vi "Motor Controller_Process.vi"(8 "error in":errorcluster, 9 "Process Sync":refnum<notifier>, 10 "TopLevel":refnum<class "TopLevel.lvclass">, 11 "Motor Controller in":refnum<class "Motor Controller.lvclass">) -> (3 "Motor Controller out":refnum<class "Motor Controller.lvclass">)   [LabVIEW 2022 SP3, in "Motor Controller.lvclass"]
uses:
  Motor Controller.lvclass
  TopLevel/TopLevel.lvclass
  Typedefs/Motor Controller Parameter-Set.ctl
  Typedefs/API Event Data.ctl
  Typedefs/API Task State.ctl
  Typedefs/API Command Cluster.ctl
  Typedefs/API Command Enum.ctl
  TopLevel/Typedefs/Motor Controller Config Data.ctl
  Typedefs/Batch Index Speed Data.ctl
  Typedefs/Move Status.ctl
  <vilib>/ethernetip/ethernetip.llb/ethernetip.ctl
  Typedefs/Motor Controller Parameter-Get.ctl
  Typedefs/SetExplicitMessage API Data.ctl
  Typedefs/StageMoves.ctl
  Typedefs/Stage Move Data.ctl
  C:/projects/Digilens_IPLC2/Classes/Motor Controller/EEIP.dll
  EEIP.dll
  <vilib>/ethernetip/ethernetip.lvlib
panel:
  out "error out":errorcluster
  in  "OK":bool
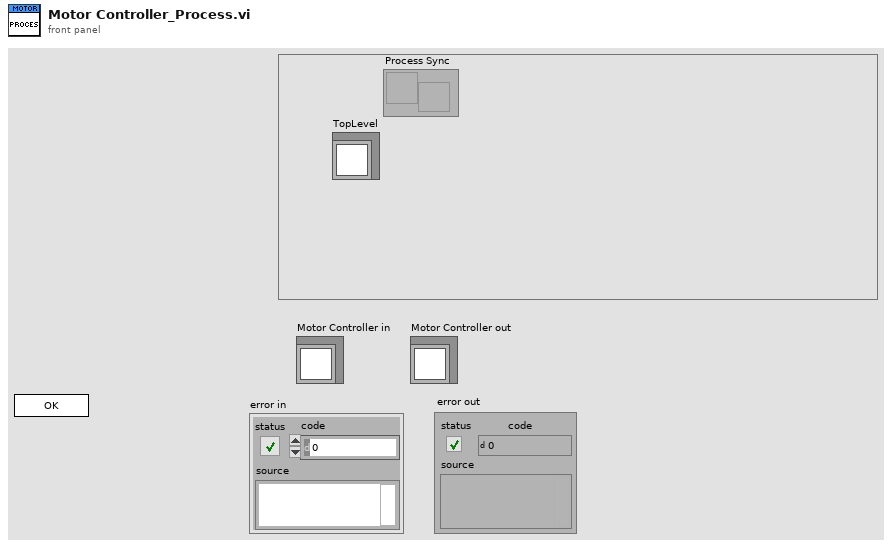
[diagram p1: front panel]
types:
  T1 = typedef "Motor Controller.lvclass/Motor Controller Parameter-Set.ctl" = enum16{"Print Speed", "Jog Speed", "PR Path", "Enable Servo", "Disable Servo", "Move Stage to Under PH1", "Move Stage to Under PH2", "Move Stage to Under PH3", "Move Stage to Under PH4", "Move Stage to Under PH5", "Move Stage to Under PH6", "Home Stage", "Return Stage to 0", "Print Stage", "Write Speed", "Write Index", "Stop Stage"}
  T2 = typedef "Motor Controller.lvclass/API Event Data.ctl" = cluster{"Task":cluster{"Time Stamp":timestamp, "Timeout (ms)":u32, "Task State":T3, "Task Error":errorcluster, "Task ID":string}, "Command":variant, "Return Value":variant}
  T3 = typedef "Motor Controller.lvclass/API Task State.ctl" = enum16{"Completed", "Errored", "Pending"}
  T4 = typedef "Motor Controller.lvclass/API Command Cluster.ctl" = cluster{"Command":T5, "Arguments":string, "Data":variant}
  T5 = typedef "Motor Controller.lvclass/API Command Enum.ctl" = enum16{"GetExplicitMessage", "SetExplicitMessage", "Execute Stage Move Recipe", "Read Stage Move Recipe", "Abort"}
  T6 = enum32{"invalid app kind", "Development System", "Run Time System", "Student Edition", "Embedded LabVIEW", "Evaluation", "Custom"}
  T7 = enum32{"Invalid", "Standard", "Closed", "Hidden", "Minimized", "Maximized"}
  T8 = typedef "Motor Controller.lvclass/Motor Controller Parameter-Get.ctl" = enum16{"Print Speed", "Jog Speed", "PR Path", "Servo Enabled?", "AlarmCodes"}
  T9 = typedef "Motor Controller.lvclass/SetExplicitMessage API Data.ctl" = cluster{"Motor Controller Parameter":T1, "value":i32}
  T10 = typedef "Motor Controller.lvclass/Stage Move Data.ctl" = cluster{"Current Step":string, "Move Data":T11[]}
  T11 = typedef "Motor Controller.lvclass/Batch Index Speed Data.ctl" = cluster{"Batch & Cycle":string, "Move":cluster{"Index_mm":i32, "Speed_mm_s":i32}, "Status":T12}
  T12 = typedef "Motor Controller.lvclass/Move Status.ctl" = enum16{"Pending", "In Progress", "Completed"}
  T13 = cluster{"Time Stamp":timestamp, "Timeout (ms)":u32, "Task State":T3, "Task Error":errorcluster, "Task ID":string}
  T14 = typedef "Motor Controller.lvclass/Motor Controller Config Data.ctl" = cluster{"Motor IP Addresss":string, "Current Position":i32, "Pulse_Per_mm":i32, "PrePrint":dbl[], "Load Position_mm":i32, "Laminate Position_mm":i32}
  T15 = typedef "TopLevel.lvclass/Digilens Config Cluster.ctl" = cluster{"Motion Controller":T14, "IO Config":T16, "PrinterConfiguration":T19, "DAQ Settings":T20}
  T16 = typedef "IO.lvclass/IO Config Data.ctl" = cluster{"DAQDevices":T17[], "DI Channels":T18[], "DO Channels":T18[], "Material Names":string[], "AI Channels":T18[], "AO Channels":T18[]}
  T17 = typedef "IO.lvclass/DCON_DeviceConfig--Cluster.ctl" = cluster{"COM":string, "DeviceName":string, "BaudRate":u32, "Number of Channels":i32, "DeviceAddress":i32, "Enable":bool}
  T18 = typedef "IO.lvclass/Channel Data.ctl" = cluster{"Channel Name":string, "Device Name":string, "Channel No":string}
  T19 = typedef "GIS Printer.lvclass/PrinterConfiguration--Cluster.ctl" = cluster{"IPAddress":string, "Move Stage on RTP Command?":bool, "Stage Move Position":string, "PH1-Prime Path":path, "PH2-Prime Path":path, "PH3-Prime Path":path, "PH4-Prime Path":path, "PH5-Prime Path":path, "PH6-Prime Path":path, "PrintScriptsFolder":path, "PurgeScriptsFolder":path, "StageScriptsFolder":path, "PH1-HeatOn Path":path, "PH2-HeatOn Path":path, "PH3-HeatOn Path":path, "PH4-HeatOn Path":path, "PH5-HeatOn Path":path, "PH6-HeatOn Path":path, "PH1-HeatOff Path":path, "PH2-HeatOff Path":path, "PH3-HeatOff Path":path, "PH4-HeatOff Path":path, "PH5-HeatOff Path":path, "PH6-HeatOff Path":path}
  T20 = typedef "DAQ.lvclass/TD DAQ Settings--cluster.ctl" = cluster{"Simulate DAQ":bool, "DI Settings":T21[], "AI Settings":T22[], "Relay IONames":string[], "AO IONames":string[], "AO NChan SingleTask":bool}
  T21 = typedef "DAQ.lvclass/TD DI Instrument Settings--cluster.ctl" = cluster{"Disable":bool, "DI TaskName":string, "DI RefreshIntv":i32}
  T22 = typedef "DAQ.lvclass/TD AI Instrument Settings--cluster.ctl" = cluster{"Disable":bool, "AI TaskName":string, "AI InstSettings":T23, "SimAI Ranges":T24}
  T23 = typedef "DAQ.lvclass/TD AI InstSettings--cluster.ctl" = cluster{"DaqRate":dbl, "NumSamples":i32}
  T24 = typedef "DAQ.lvclass/TD SimAI Ranges--cluster.ctl" = cluster{"lo":dbl, "hi":dbl}
  T25 = typedef "ethernetip.lvlib/ethernetip.ctl" = refnum<k21>
  T26 = cluster{"Core":cluster{"Current VI Reference":refnum<vi>, "Close Panel on Exit?":bool}, "Motor Controller out":refnum<class "Motor Controller.lvclass">, "Tasks":T2[], "TO":i32, "API Executed Event":refnum<user-event>, "API Return Event":refnum<user-event>, "Current Task":T4, "Task Start ms":u32, ".NET Refnum":refnum<k24>, "Current Task. Return Value":variant, "Motion Controller Config Data":T14, "Methods:Accessors:Digilens Config":T15, "Stage Moves":T11[], "Move Index":i32, "Session out":T25, "Process Sync":refnum<notifier>}
  T27 = cluster{"Current VI Reference":refnum<vi>, "Close Panel on Exit?":bool}
  T28 = typedef "Motor Controller.lvclass/UserEvents.ctl" = cluster{"API Incoming Event":refnum<user-event>, "API Executed Event":refnum<user-event>, "API Return Event":refnum<user-event>, "Status Changed Event":refnum<user-event>, "StopEvent":refnum<user-event>}
  T29 = typedef "TopLevel.lvclass/UserEvents.ctl" = cluster{"API Incoming Event":refnum<user-event>, "API Executed Event":refnum<user-event>, "API Return Event":refnum<user-event>, "Exit Event":refnum<user-event>, "StatusChanged":refnum<user-event>, "DLP GUI Config Changed":refnum<user-event>, "AppEvent":refnum<user-event>, "Login Event":refnum<user-event>, "HeadPrimeStatusEvent":refnum<user-event>}
  T30 = typedef "Motor Controller.lvclass/StageMoves.ctl" = cluster{"Batch_Move":cluster{"Cycles":u32, "Move":cluster{"Index_mm":i32, "Speed_mm_s":i32}[]}[]}
  T31 = cluster{"Cycles":u32, "Move":cluster{"Index_mm":i32, "Speed_mm_s":i32}[]}[]
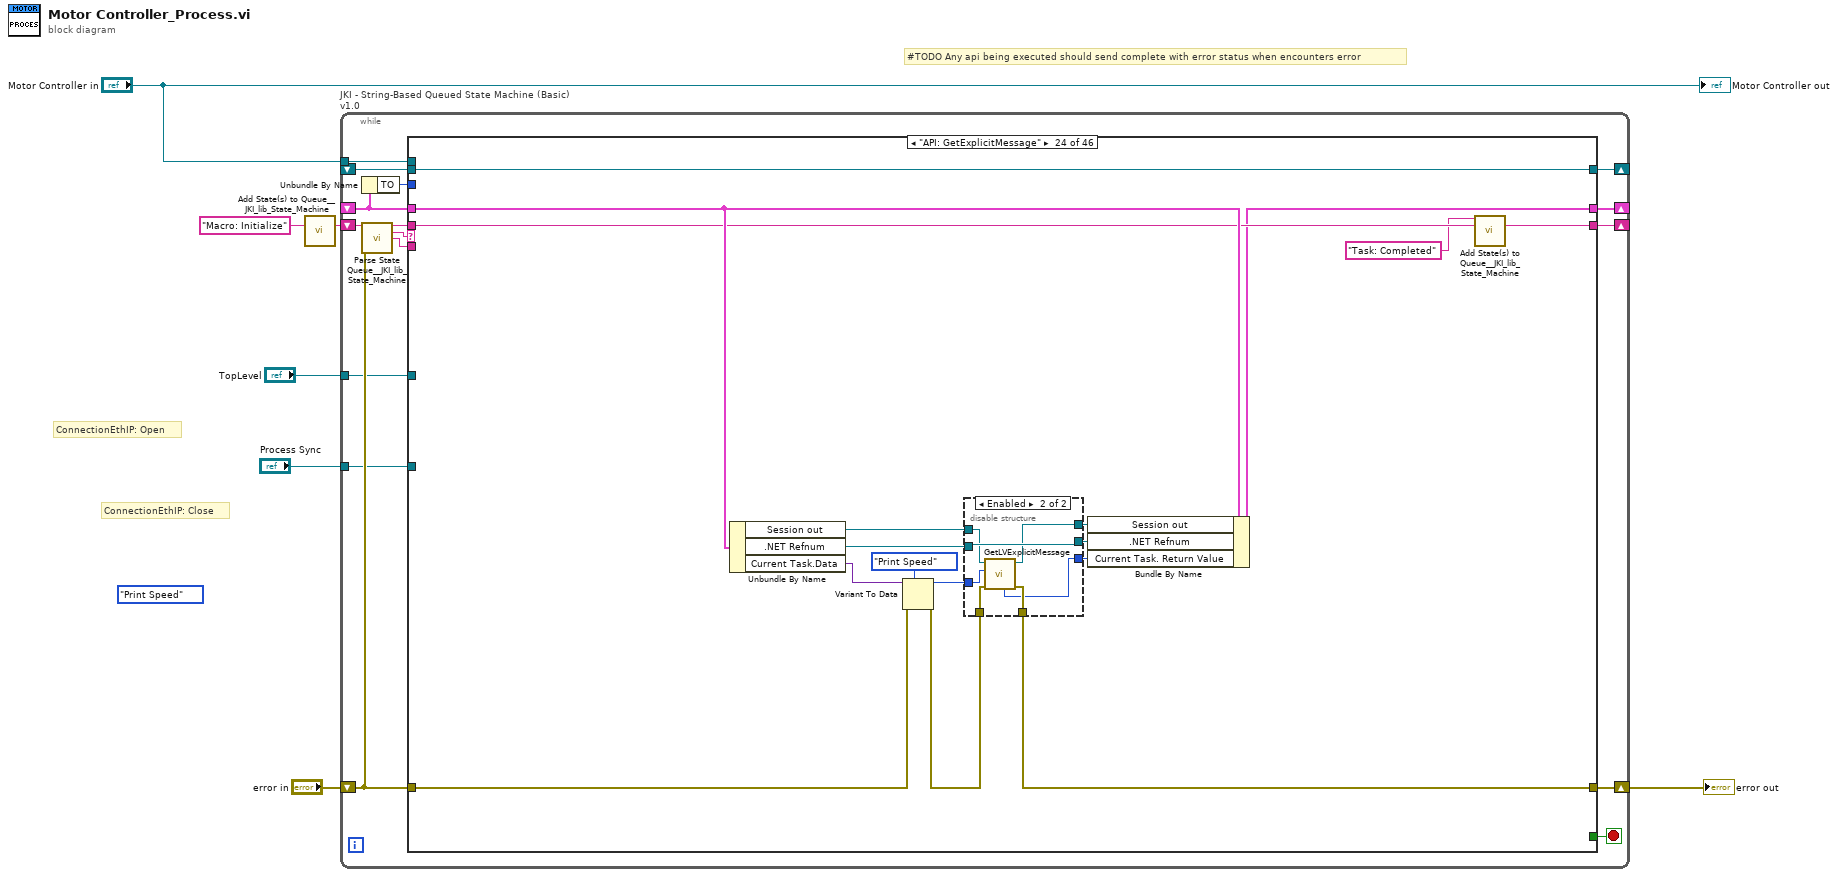
[diagram p0: block diagram]
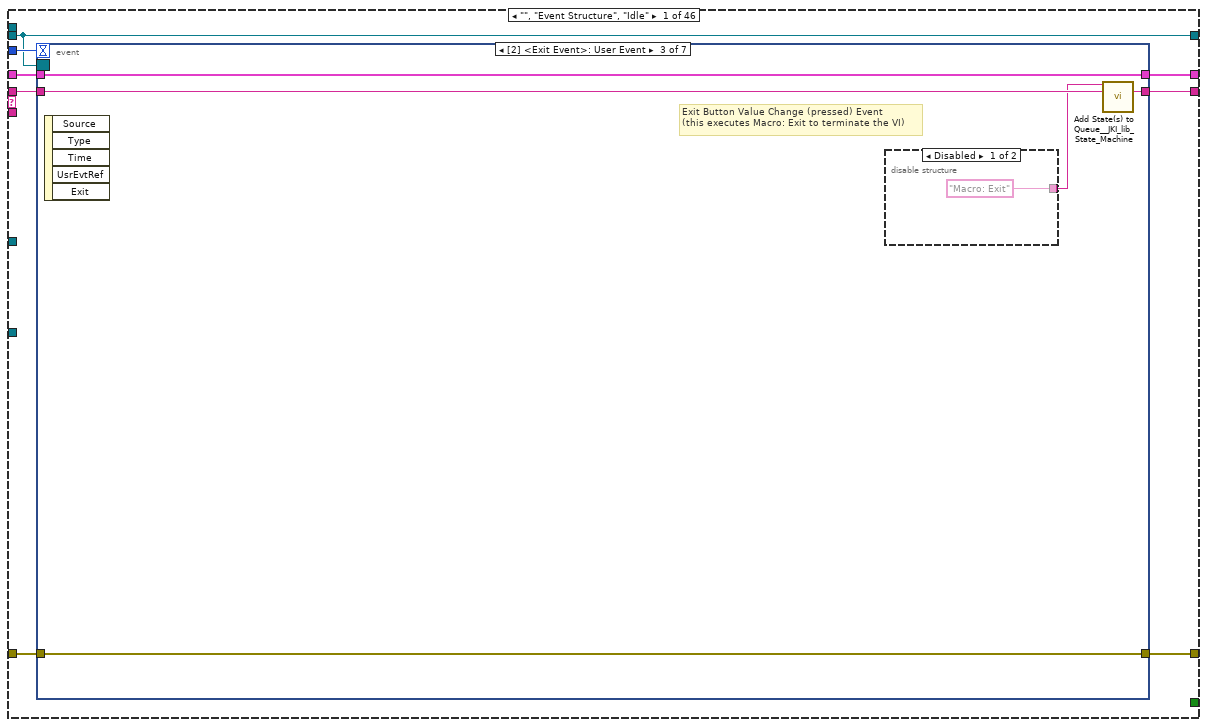
[diagram p2: hidden frame]
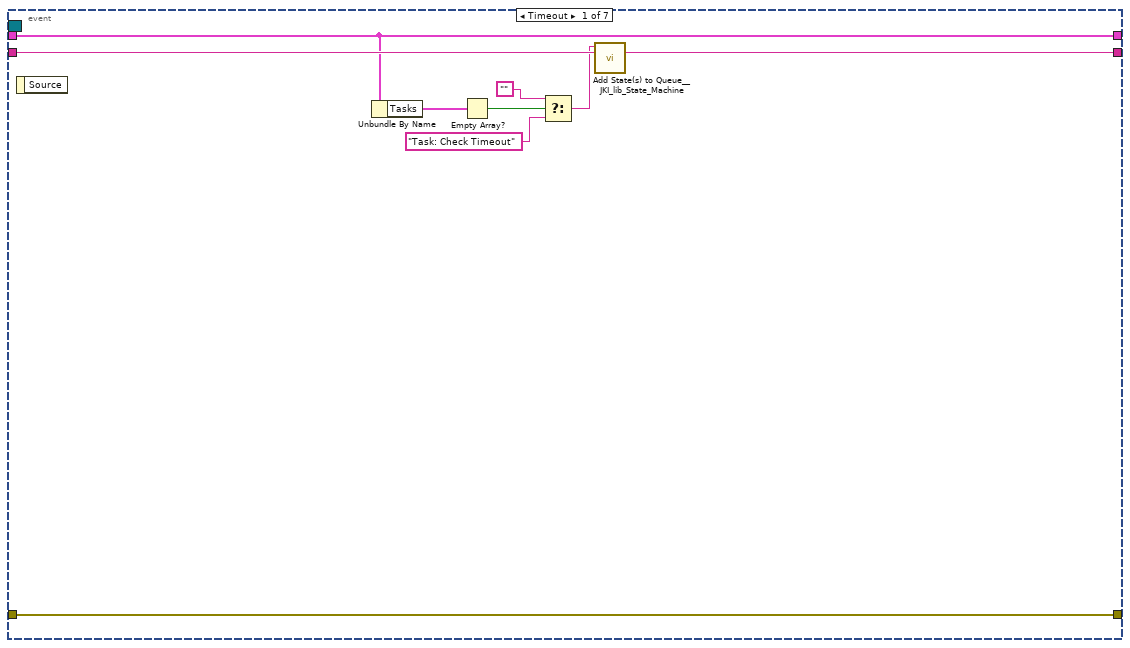
[diagram p3: hidden frame]
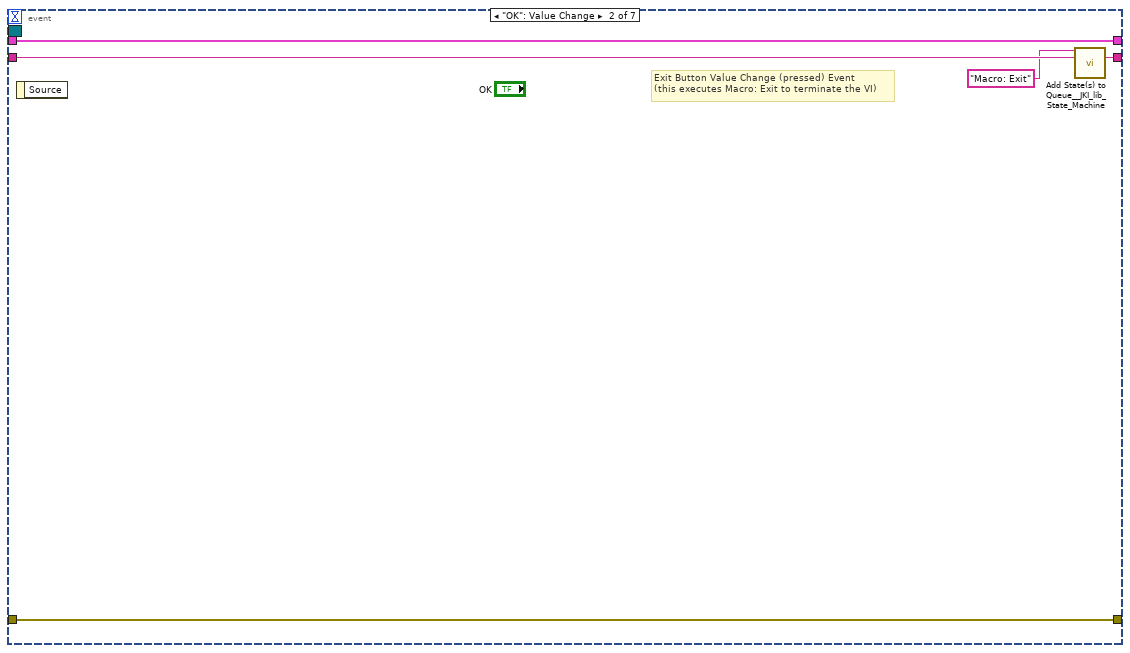
[diagram p4: hidden frame]
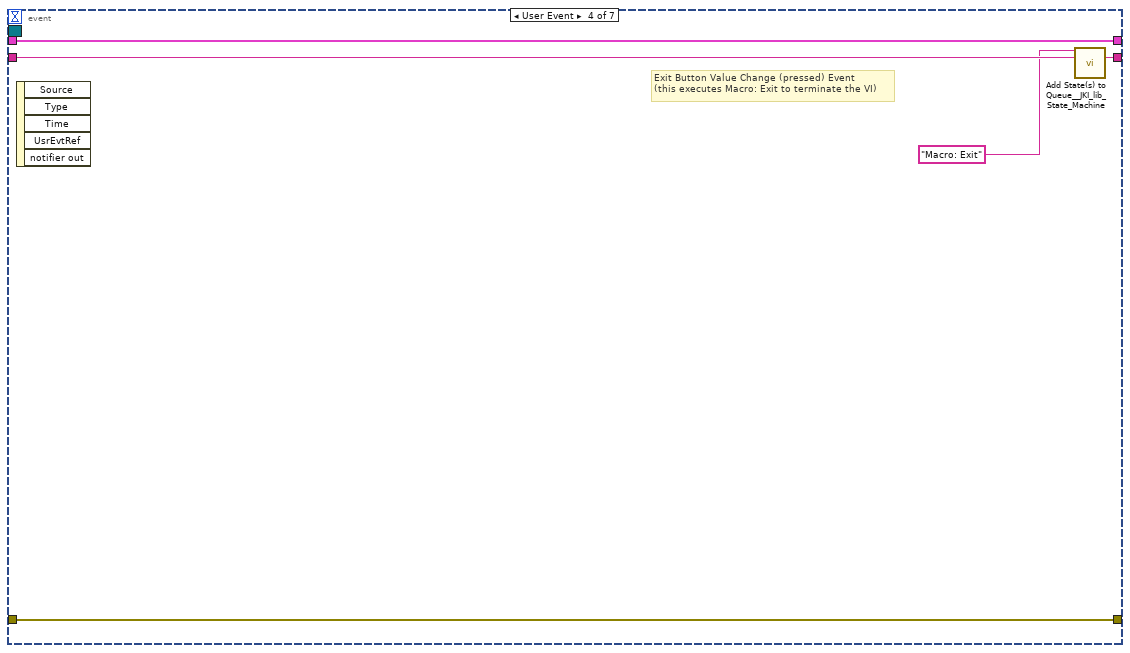
[diagram p6: hidden frame]
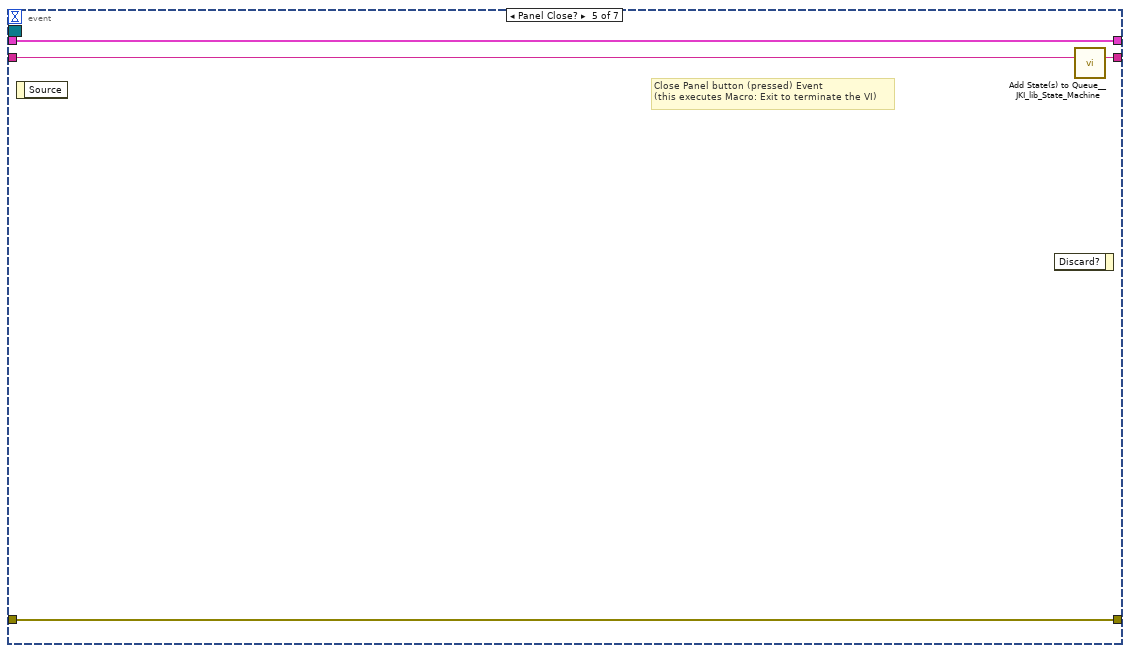
[diagram p7: hidden frame]
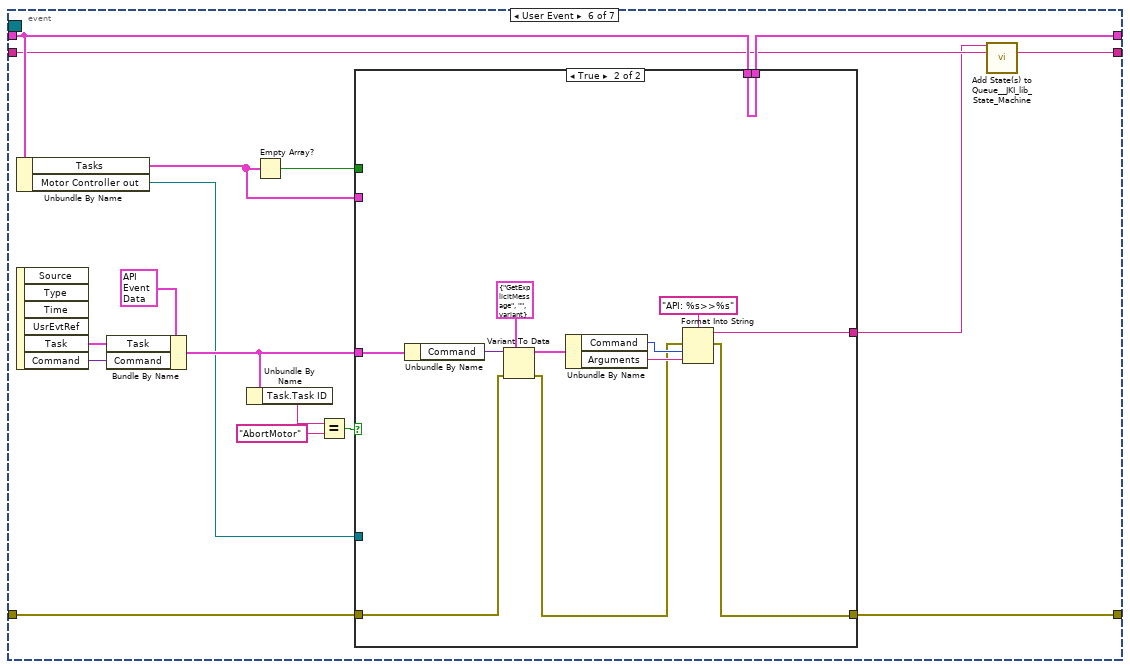
[diagram p8: hidden frame]
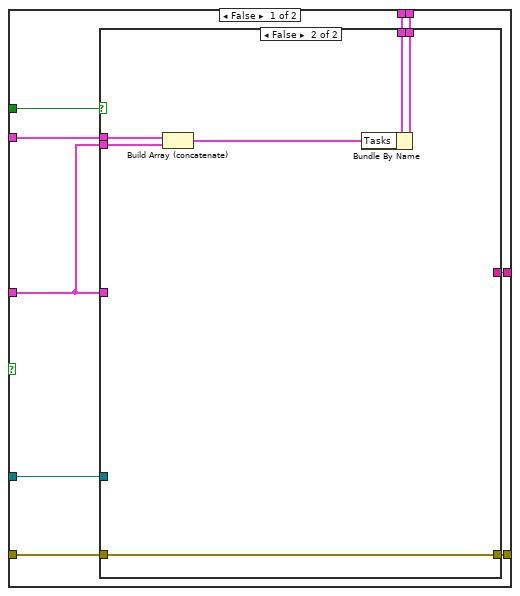
[diagram p9: hidden frame]
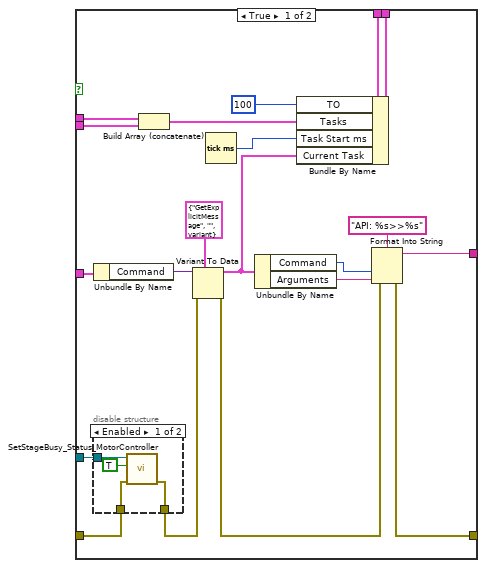
[diagram p10: hidden frame]
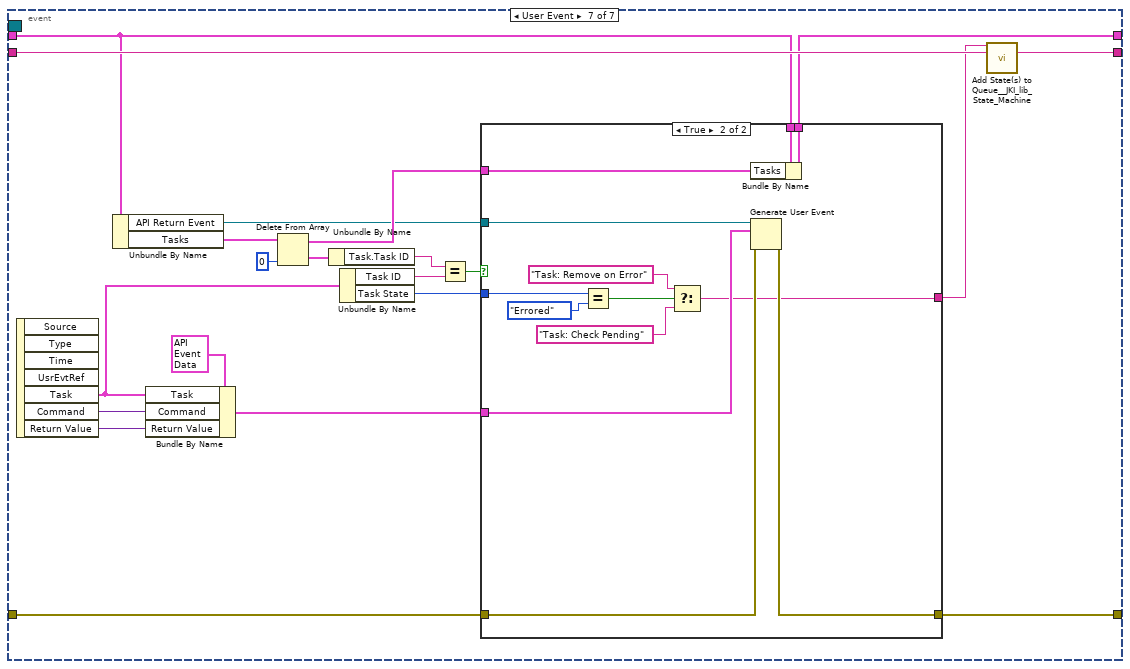
[diagram p12: hidden frame]
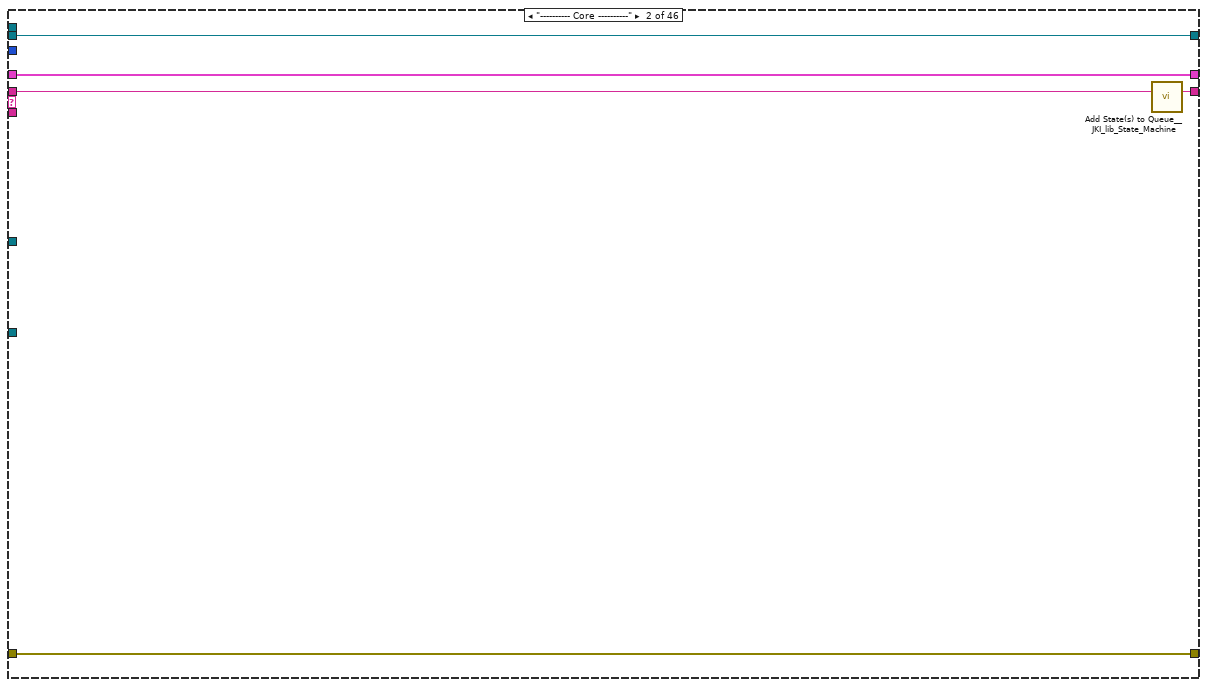
[diagram p14: hidden frame]
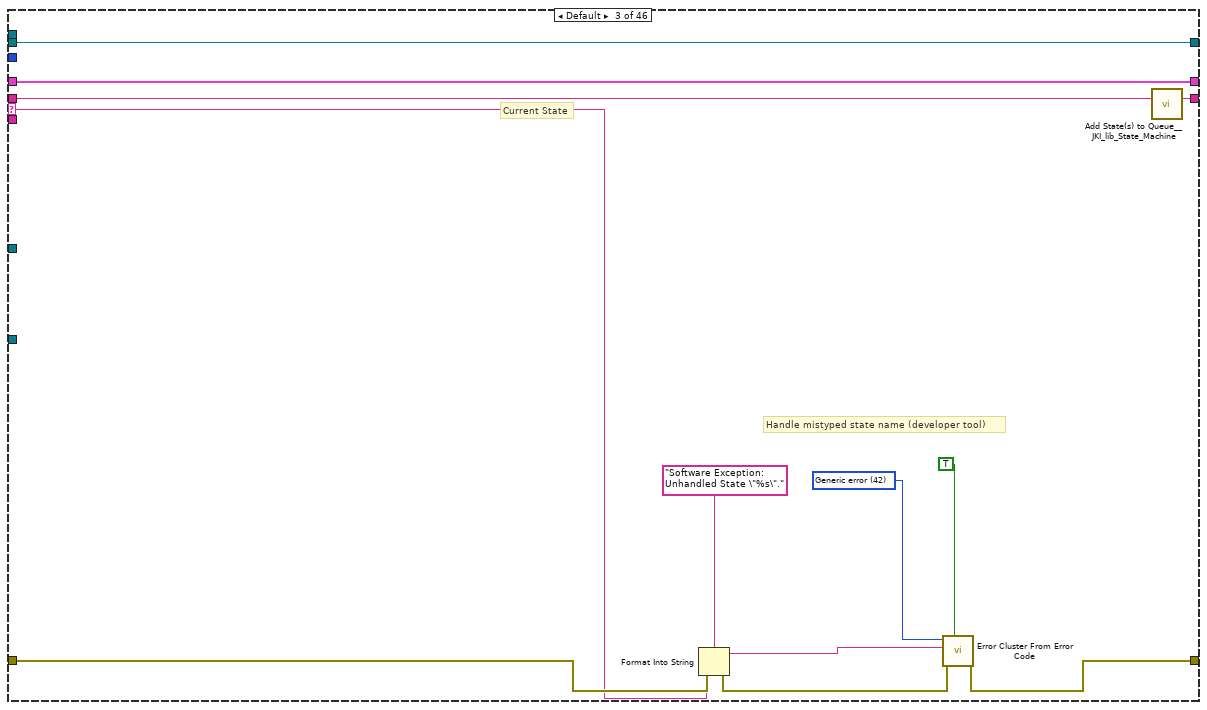
[diagram p15: hidden frame]
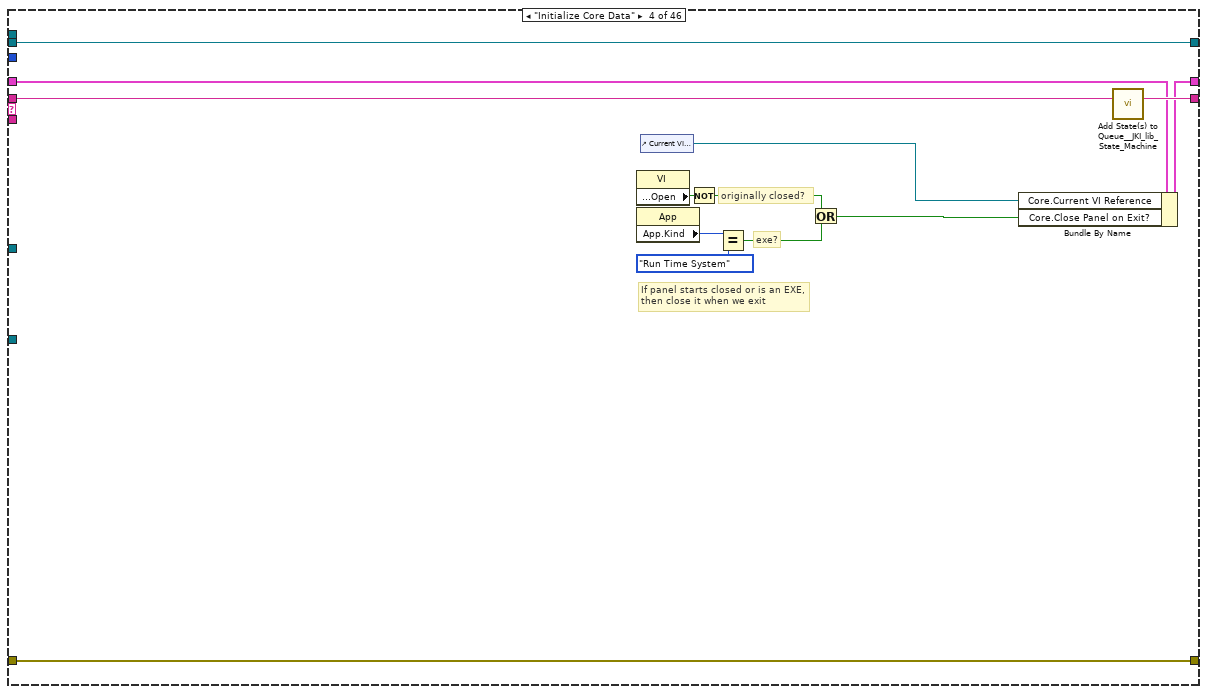
[diagram p16: hidden frame]
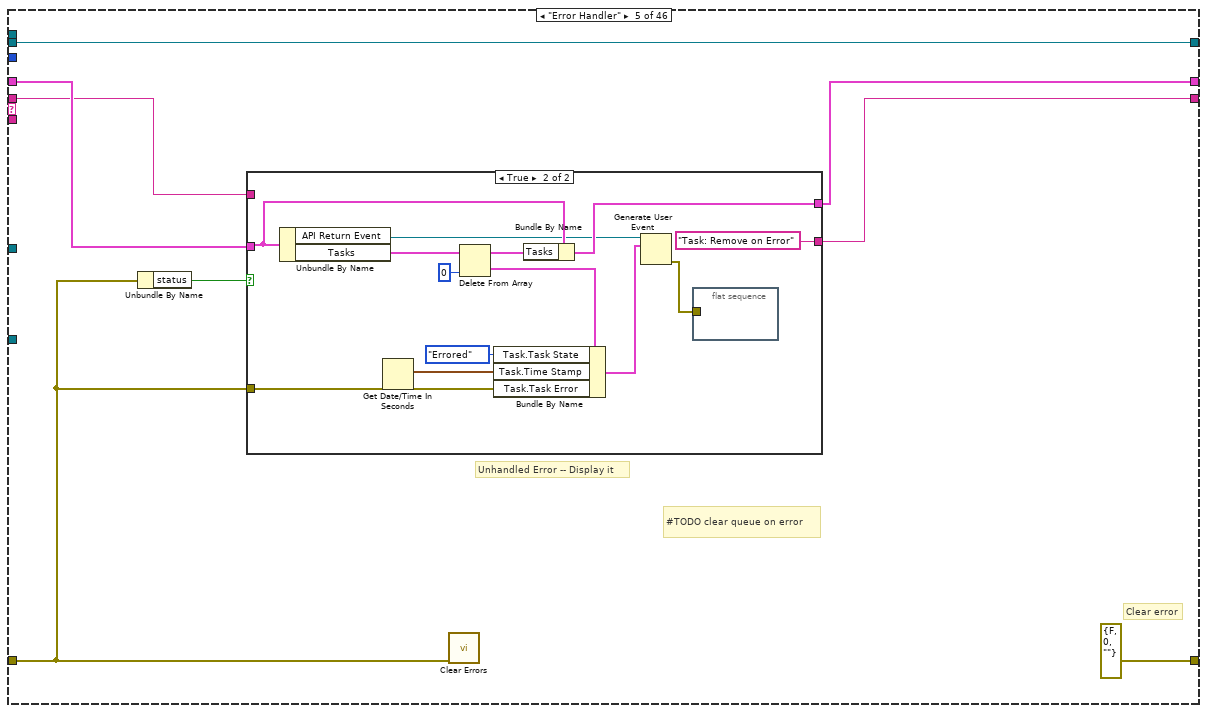
[diagram p17: hidden frame]
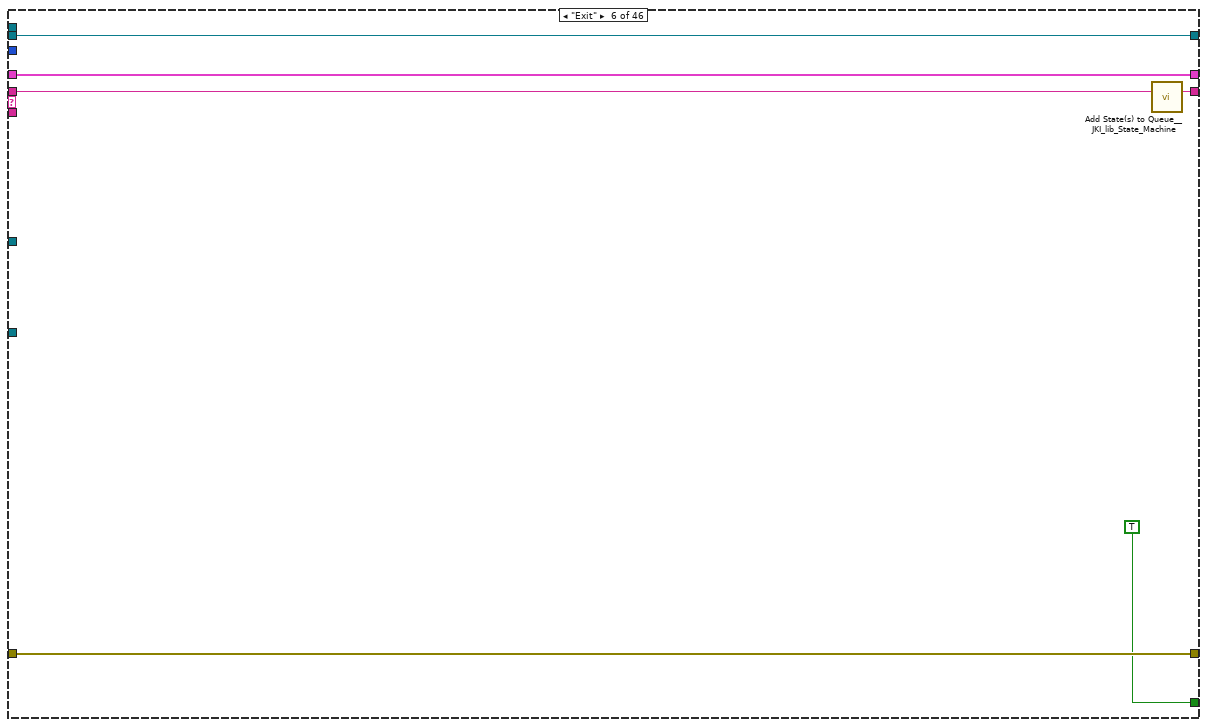
[diagram p19: hidden frame]
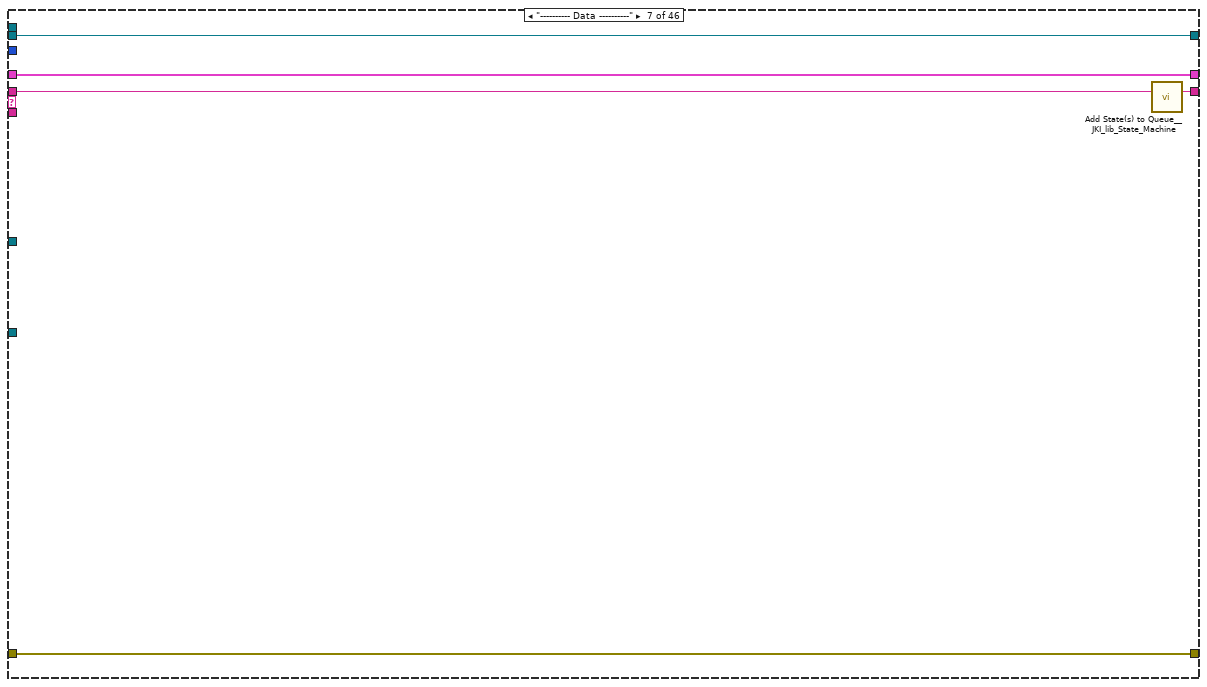
[diagram p20: hidden frame]
diagram:
  (unwired) Motor_Controller_Parameter-Set."Print Speed" ("Motor Controller Parameter")
  # "ConnectionEthIP: Close"
  # "ConnectionEthIP: Open"
  # "#TODO Any api being executed should send complete with error status when encounters error"
  n1 = call <vilib>:"Add State(s) to Queue__JKI_lib_State_Machine.vi"("State(s) in (\"\")"="Macro: Initialize") -> ("States Out"=w7:string)  [unwired: 14 in]
  n2 = while "JKI - String-Based Queued State Machine (Basic) v1.0" {
    shift-right: [w16] -> _
    shift-left: _ -> [w10]
    shift-right: [w19] -> w3
    shift-left: "error in" -> [w15]
    shift-right: [w18] -> _
    shift-left: w7 -> [w20]
    tunnel: "Motor Controller in" -> [w14]
    shift-right: [w13] -> _
    shift-left: _ -> [w12]
    tunnel: "TopLevel" -> [w9]
    tunnel: "Process Sync" -> [w8]
    stop <- w17 stop-if-true
    n3 = Unbundle By Name(w10) -> ("TO"=w11:i32)
    n4 = call <vilib>:"Parse State Queue__JKI_lib_State_Machine.vi"("State Queue"=w20, "Error In (no error)"=w15) -> ("Remaining States"=w22:string, "Current State"=w23:string, "Arguments"=w21:string)  [unwired: 11 in]
    n5 = case shown="\"API: GetExplicitMessage\"" w23 {
      selector: w23 -> [_ _ w172 _ _ _ _ _ _ _ _ _ _ _ _ _ _ _ _ _ _ _ _ _ _ _ _ _ _ _ _ _ _ _ _ _ _ _ _ _ _ _ _ _ _ _]
      tunnel: w22 -> [w31 w170 w176 w195 w196 w224 w229 w237 w263 w272 w277 w283 w290 w302 w329 _ w345 w347 w355 w371 w377 w379 _ w398 w435 w475 w500 w512 w520 w531 w551 w580 w624 w641 w650 w656 w664 w671 w674 w686 w700 w703 w773 w859 w866 w895]
      tunnel: w21 -> [_ _ _ _ _ _ _ _ _ _ _ _ w285 w296 _ _ _ _ _ _ _ _ _ _ _ _ _ _ _ _ _ _ _ _ _ _ _ _ _ _ _ w721 _ _ _ _]
      tunnel: w10 -> [w29 w167 w174 w186 w198 w222 w226 w234 _ w268 w274 w281 w288 w298 w326 w331 w342 w350 w353 w368 w375 w380 w383 w407 w441 w479 w505 w517 w521 w529 w549 w577 w621 w640 w643 w653 w663 w667 w673 w684 w699 w709 w771 w857 w878 w897]
      tunnel: [w28 w168 w178 w192 errorcluster {"status"=FALSE, "code"=0, "source"=""} ("error out") w221 w227 w231 w244 w269 w275 w278 w286 w299 w327 w334 w343 w351 w354 w366 w373 w378 w387 w405 w426 w469 w496 w508 w519 w525 w546 w585 w615 w642 w646 w652 w660 w668 w675 w682 w701 w711 w749 w849 w875 w904] -> w19
      tunnel: w15 -> [w27 w168 w177 w192 w200 w221 w227 w230 w257 w264 w275 w279 w287 w300 w327 w334 w343 w351 w354 w361 w374 w378 w388 w400 w437 w477 w503 w515 w519 w524 w545 w584 w620 w642 w645 w651 w665 w669 w675 w681 w701 w719 w755 w850 w874 w904]
      tunnel: [w30 w169 w175 w194 w197 w223 w228 w236 w263 w271 w276 w282 w289 w301 w328 w333 w344 w348 w355 w370 w376 w379 "Task: Remove on Error" ("State(s) at Back (\"\")") w399 w436 w476 w501 w513 w520 w531 w551 w581 w625 w641 w650 w656 w664 w671 w674 w686 w700 w704 w773 w859 w867 w896] -> w18
      tunnel: [_ _ _ _ _ TRUE _ _ _ _ _ _ _ _ _ _ _ _ _ _ _ _ _ _ _ _ _ _ _ _ _ _ _ _ _ _ _ _ _ _ _ _ _ _ _ _] -> w17
      tunnel: [w26 w167 w174 w193 w199 w222 w226 w234 w262 w268 w274 w281 w288 w298 w326 w331 w342 w350 w353 w358 w375 w380 w384 w396 w434 w474 w505 w517 w521 w529 w549 w578 w619 w640 w644 w653 w658 w667 w673 w677 w699 w710 w758 w852 w878 w898] -> w16
      tunnel: w11 -> [w25 _ _ _ _ _ _ _ _ _ _ _ _ _ _ _ _ _ _ _ _ _ _ _ _ _ _ _ _ _ _ _ _ _ _ _ _ _ _ _ _ _ _ _ _ _]
      tunnel: w14 -> [_ _ _ _ _ _ _ _ w239 _ _ _ _ _ _ _ _ _ _ _ _ _ _ _ _ _ _ _ _ _ _ _ _ _ _ _ _ _ _ _ _ _ _ _ _ _]
      tunnel: [w24 w166 w171 w183 w202 w219 w225 w235 w260 w267 w273 w280 w284 w295 w325 w330 w335 w349 w352 w369 w372 w381 w391 w408 w442 w480 w506 w518 w522 w530 w550 w588 w626 w639 w649 w655 w662 w670 w672 w685 w698 w722 w772 w858 w879 w903] -> w13
      tunnel: w12 -> [w24 w166 w171 w183 w202 w219 w225 w235 w260 w267 w273 w280 w284 w295 w325 w330 w335 w349 w352 _ w372 w381 w391 w408 w442 w480 w506 w518 w522 w530 w550 w588 w626 w639 w649 w655 w662 w670 w672 w685 w698 w722 w772 w858 w879 w903]
      tunnel: w9 -> [_ _ _ _ _ _ _ _ w242 _ _ _ _ _ _ _ _ _ _ w363 _ _ _ _ _ _ _ _ _ _ _ _ _ _ _ _ _ _ _ _ _ _ _ _ _ _]
      tunnel: w8 -> [_ _ _ _ _ _ _ _ w238 _ _ _ _ _ _ _ _ _ _ _ _ _ _ _ _ _ _ _ _ _ _ _ _ _ _ _ _ _ _ _ _ _ _ _ _ _]
      frame "", "Event Structure", "Idle" {
        n6 = event shown="[2] <Exit Event>: User Event" {
          selector: w24 -> [_ _ _ _ _ _ _]
          dyn-events: _ -> [_ _ _ _ _ _ _]
          timeout: w25 -> [_ _ _ _ _ _ _]
          tunnel: w31 -> [w40 w45 w50 w56 w60 w67 w149]
          tunnel: [w39 w44 w49 w55 w59 w68 w150] -> w30
          tunnel: w29 -> [w37 w42 w47 w53 w57 w71 w148]
          tunnel: [w38 w43 w48 w54 w58 w70 w142] -> w28
          tunnel: w27 -> [w38 w43 w48 w54 w58 w69 w143]
          tunnel: [w37 w42 w47 w53 w57 w72 w145] -> w26
          event Timeout {
            n7 = event-data() -> ()  [unwired: 1 in, 1 out]
            n8 = Unbundle By Name(w37) -> ("Tasks"=w36:T2[])
            n9 = Empty Array?(array=w36) -> (empty?=w35:bool)
            n10 = Select(t="", s=w35, f="Task: Check Timeout") -> (s? t:f=w32:string)
            n11 = call <vilib>:"Add State(s) to Queue__JKI_lib_State_Machine.vi"("State(s) in Front (\"\")"=w32, "State(s) in (\"\")"=w40) -> ("States Out"=w39:string)  [unwired: 13 in]
          }
          event "OK": Value Change {
            # "Exit Button Value Change (pressed) Event\n(this executes Macro: Exit to terminate the VI)"
            n12 = event-data() -> ()  [unwired: 1 in, 1 out]
            n13 = call <vilib>:"Add State(s) to Queue__JKI_lib_State_Machine.vi"("State(s) in Front (\"\")"="Macro: Exit", "State(s) in (\"\")"=w45) -> ("States Out"=w44:string)  [unwired: 13 in]
          }
          event User Event {
            # "Exit Button Value Change (pressed) Event\n(this executes Macro: Exit to terminate the VI)"
            n14 = event-data() -> ()  [unwired: 1 in, 5 out]
            n15 = disable-structure shown="Disabled" {
              disable-tunnel: ["Macro: Exit" _] -> w46
              frame Disabled {
              }
              frame Enabled {
              }
            }
            n16 = call <vilib>:"Add State(s) to Queue__JKI_lib_State_Machine.vi"("State(s) in Front (\"\")"=w46, "State(s) in (\"\")"=w50) -> ("States Out"=w49:string)  [unwired: 13 in]
          }
          event User Event {
            # "Exit Button Value Change (pressed) Event\n(this executes Macro: Exit to terminate the VI)"
            n17 = event-data() -> ()  [unwired: 1 in, 5 out]
            n18 = call <vilib>:"Add State(s) to Queue__JKI_lib_State_Machine.vi"("State(s) in Front (\"\")"="Macro: Exit", "State(s) in (\"\")"=w56) -> ("States Out"=w55:string)  [unwired: 13 in]
          }
          event Panel Close? {
            # "Close Panel button (pressed) Event\n(this executes Macro: Exit to terminate the VI)"
            n19 = event-data() -> ()  [unwired: 1 in, 1 out]
            n20 = event-data() -> ()  [unwired: 2 in, 1 out]
            n21 = call <vilib>:"Add State(s) to Queue__JKI_lib_State_Machine.vi"("State(s) in (\"\")"=w60) -> ("States Out"=w59:string)  [unwired: 14 in]
          }
          event User Event {
            n22 = Unbundle By Name(w71) -> ("Tasks"=w73:T2[], "Motor Controller out"=w61:refnum<class "Motor Controller.lvclass">)
            n23 = event-data() -> ("Task"=w76:T13, "Command"=w75:variant)  [unwired: 1 in, 4 out]
            n24 = Bundle By Name(cluster=T2 {"Task"={"Time Stamp"=timestamp(0 s since 1904-01-01), "Timeout (ms)"=0, "Task State"=enum."Completed", "Task Error"={"status"=FALSE, "code"=0, "source"=""}, "Task ID"=""}, "Command"=variant, "Return Value"=variant} ("API Event Data"), "Task"=w76, "Command"=w75) -> (w65:T2)
            n25 = Unbundle By Name(w65) -> ("Task.Task ID"=w64:string)
            n26 = Empty Array?(array=w73) -> (empty?=w74:bool)
            n27 = Equal?(x=w64, y="AbortMotor") -> (x = y?=w62:bool)
            n28 = case shown="True" w62 {
              tunnel: w74 -> [w86 _]
              tunnel: w73 -> [w85 _]
              tunnel: [w84 w129] -> w72
              tunnel: w71 -> [w83 w129]
              tunnel: [w82 w118] -> w70
              tunnel: w69 -> [w81 w120]
              tunnel: [w80 w121] -> w66
              tunnel: w65 -> [w79 w122]
              tunnel: w61 -> [w78 _]
              frame False {
                n29 = case shown="False" w86 {
                  tunnel: w85 -> [w106 w117]
                  tunnel: w79 -> [w105 w116]
                  tunnel: w83 -> [w104 w115]
                  tunnel: [w102 w113] -> w84
                  tunnel: w79 -> [w101 _]
                  tunnel: w81 -> [w87 w112]
                  tunnel: [w97 w112] -> w82
                  tunnel: [w94 _] -> w80
                  tunnel: w78 -> [w89 _]
                  frame True {
                    n30 = Unbundle By Name(w101) -> ("Command"=w100:variant)
                    n31 = disable-structure shown="Enabled" {
                      disable-tunnel: w89 -> [w110 _]
                      disable-tunnel: [w108 w111] -> w88
                      disable-tunnel: w87 -> [w107 w111]
                      frame Enabled {
                        n32 = call "SetStageBusy_Status_MotorController.vi"("error in (no error)"=w107, "Stage Busy?"=TRUE, "Motor Controller in"=w110) -> ("error out"=w108:errorcluster)  [unwired: 7 in, 1 out]
                      }
                      frame Disabled {
                      }
                    }
                    n33 = Build Array (concatenate)(w106, w105) -> (w103:T2[])
                    n34 = Variant To Data(error in=w88, type=T4 {"Command"=enum."GetExplicitMessage", "Arguments"="", "Data"=variant} ("API Command Cluster"), Variant=w100) -> (data=w90:T4, error out=w98:errorcluster)
                    n35 = Tick Count (ms)() -> (millisecond timer value=w92:u32)
                    n36 = Unbundle By Name(w90) -> ("Command"=w95:T5, "Arguments"=w93:string)
                    n37 = Bundle By Name(cluster=w104, "TO"=100, "Tasks"=w103, "Task Start ms"=w92, "Current Task"=w90) -> (w102:T26)
                    n38 = Format Into String(format string="API: %s>>%s", error in=w98, w95, w93) -> (resulting string=w94:string, error out=w97:errorcluster)  [unwired: 1 in]
                  }
                  frame False {
                    n39 = Build Array (concatenate)(w117, w116) -> (w114:T2[])
                    n40 = Bundle By Name(cluster=w115, "Tasks"=w114) -> (w113:T26)
                  }
                }
              }
              frame True {
                n41 = Unbundle By Name(w122) -> ("Command"=w128:variant)
                n42 = Variant To Data(error in=w120, type=T4 {"Command"=enum."GetExplicitMessage", "Arguments"="", "Data"=variant} ("API Command Cluster"), Variant=w128) -> (data=w123:T4, error out=w119:errorcluster)
                n43 = Unbundle By Name(w123) -> ("Command"=w125:T5, "Arguments"=w124:string)
                n44 = Format Into String(format string="API: %s>>%s", error in=w119, w125, w124) -> (resulting string=w121:string, error out=w118:errorcluster)  [unwired: 1 in]
              }
            }
            n45 = call <vilib>:"Add State(s) to Queue__JKI_lib_State_Machine.vi"("State(s) in Front (\"\")"=w66, "State(s) in (\"\")"=w67) -> ("States Out"=w68:string)  [unwired: 13 in]
          }
          event User Event {
            n46 = event-data() -> ("Task"=w136:T13, "Command"=w140:variant, "Return Value"=w139:variant)  [unwired: 1 in, 4 out]
            n47 = Unbundle By Name(w148) -> ("API Return Event"=w133:refnum<user-event>, "Tasks"=w147:T2[])
            n48 = Bundle By Name(cluster=T2 {"Task"={"Time Stamp"=timestamp(0 s since 1904-01-01), "Timeout (ms)"=0, "Task State"=enum."Completed", "Task Error"={"status"=FALSE, "code"=0, "source"=""}, "Task ID"=""}, "Command"=variant, "Return Value"=variant} ("API Event Data"), "Task"=w136, "Command"=w140, "Return Value"=w139) -> (w138:T2)
            n49 = Delete From Array(array=w147, index=0) -> (deleted portion=w137:T2, array with subset deleted=w144:T2[])  [unwired: 1 in]
            n50 = Unbundle By Name(w137) -> ("Task.Task ID"=w135:string)
            n51 = Unbundle By Name(w136) -> ("Task ID"=w134:string, "Task State"=w131:T3)
            n52 = Equal?(x=w135, y=w134) -> (x = y?=w132:bool)
            n53 = case shown="True" w132 {
              tunnel: w148 -> [w152 w165]
              tunnel: [w152 w164] -> w145
              tunnel: w144 -> [_ w163]
              tunnel: w133 -> [_ w162]
              tunnel: w143 -> [w151 w159]
              tunnel: [w151 w160] -> w142
              tunnel: w138 -> [_ w161]
              tunnel: w131 -> [_ w158]
              tunnel: [_ w153] -> w130
              frame False {
              }
              frame True {
                n54 = Equal?(x=w158, y=API_Task_State."Errored") -> (x = y?=w156:bool)
                n55 = Select(t="Task: Remove on Error", s=w156, f="Task: Check Pending") -> (s? t:f=w153:string)
                n56 = Bundle By Name(cluster=w165, "Tasks"=w163) -> (w164:T26)
                n57 = Generate User Event(user event=w162, event data cluster=w161, error in=w159) -> (error out=w160:errorcluster)  [unwired: 1 in, 1 out]
              }
            }
            n58 = call <vilib>:"Add State(s) to Queue__JKI_lib_State_Machine.vi"("State(s) in Front (\"\")"=w130, "State(s) in (\"\")"=w149) -> ("States Out"=w150:string)  [unwired: 13 in]
          }
        }
      }
      frame "---------- Core ----------" {
        n59 = call <vilib>:"Add State(s) to Queue__JKI_lib_State_Machine.vi"("State(s) in (\"\")"=w170) -> ("States Out"=w169:string)  [unwired: 14 in]
      }
      frame Default {
        w181 = 42 items=["No error", "Argument error", "Memory is full", "Out of zone", "End of file", "File already open", "Generic file I/O error", "File not found", "File permission error", "Disk is full", "Duplicate path", "Too many files open", "System feature not enabled", "Resource file not found", "Cannot add resource", "Resource not found", "Image not found", "Image memory error", "Pen does not exist", "Config type invalid", "Config token not found", "Config parse error", "Config memory error", "Bad external code format", "Bad external code offset", "External code not present", "Null window", "Destroy window error", "Null menu", "Print aborted", "Bad print record", "Print driver error", "Windows error during printing", "Memory error during printing", "Print dialog error", "Generic print error", "Invalid device refnum", "Device not found", "Device parameter error", "Device unit error", "Cannot open device", "Device call aborted", "Generic error", "Cancelled by user", "Object ID too low", "Object ID too high", "Object not in heap", "Unknown heap", "Unknown object (invalid DefProc)", "Unknown object (DefProc not in table)", "Message out of range", "Invalid (null) method", "Unknown message", "Manager call not supported", "Bad address", "Network operation in progress", "Network operation timed out", "Connection is busy", "Network attribute not supported", "Network error", "Address in use", "System out of memory", "Connection aborted", "Connection refused", "Not connected", "Already connected", "Connection closed", "Initialization error (interapplication manager)", "Bad occurrence", "Wait on unbound occurrence handler", "Occurrence queue overflow", "Datalog type conflict", "Unused", "Unrecognized type (interapplication manager)", "Memory corrupt", "Failed to make temporary DLL", "Old CIN version", "Drag socket not found", "Failed to load drop-object", "Failed to register OLE object", "Failed to release OLE object", "Format specifier type mismatch", "Unknown format specifier", "Too few format specifiers", "Too many format specifiers", "Scan failed", "Newer CIN version", "Error converting to variant", "Runtime menu error", "Password tampered", "Variant attribute not found", "Incompatible variant data type", "Event data is not available", "Event Store is not present", "Occurrence is not found", "Event Queue is not created", "Event info is not available", "Refnum passed is NULL", "Error retrieving Class GUID", "Error retrieving CoClass GUID", "Error retrieving TypeLib GUID.", "Bad built application magic bytes.", "Specific driver is different from the specific driver associated with the Logical Name.", "There is no session opened to the class driver.", "Max Error", "MAX - Error with config objects", "MAX - Error loading configuration", "MAX - Group not supported"]
        # "Current State"
        # "Handle mistyped state name (developer tool)"
        n60 = Format Into String(format string="Software Exception: Unhandled State \"%s\"." ("message"), error in=w177, w172) -> (resulting string=w180:string, error out=w179:errorcluster)  [unwired: 1 in]
        n61 = call <vilib>:"Error Cluster From Error Code.vi"("show call chain? (False)"=TRUE, "error in (no error)"=w179, "error message (\"\")"=w180, "error code (0)"=w181) -> ("error out"=w178:errorcluster)  [unwired: 5 in]
        n62 = call <vilib>:"Add State(s) to Queue__JKI_lib_State_Machine.vi"("State(s) in (\"\")"=w176) -> ("States Out"=w175:string)  [unwired: 14 in]
      }
      frame "Initialize Core Data" {
        # "originally closed?"
        # "exe?"
        # "If panel starts closed or is an EXE, then close it when we exit"
        n63 = property class="VI"() -> ("Front Panel.Open"=w191:bool)  [unwired: 2 in, 2 out]
        n64 = property class="App"() -> ("App.Kind"=w190:T6)  [unwired: 2 in, 2 out]
        n65 = control-ref of="Current VI Reference"() -> (w184:refnum<vi>)
        n66 = Not(x=w191) -> (.not. x?=w188:bool)
        n67 = Equal?(x=w190, y=T6."Run Time System" ("Application:Kind")) -> (x = y?=w187:bool)
        n68 = Or(x=w188, y=w187) -> (x .or. y?=w185:bool)
        n69 = Bundle By Name(cluster=w186, "Core.Current VI Reference"=w184, "Core.Close Panel on Exit?"=w185) -> (w193:T26)
        n70 = call <vilib>:"Add State(s) to Queue__JKI_lib_State_Machine.vi"("State(s) in (\"\")"=w195) -> ("States Out"=w194:string)  [unwired: 14 in]
      }
      frame "Error Handler" {
        # "#TODO clear queue on error"
        # "Unhandled Error -- Display it"
        # "Clear error"
        n71 = Unbundle By Name(w200) -> ("status"=w201:bool)
        n72 = case shown="True" w201 {
          tunnel: w198 -> [w205 w216]
          tunnel: [w205 w214] -> w199
          tunnel: w200 -> [_ w209]
          tunnel: [w204 "Task: Remove on Error"] -> w197
          tunnel: w196 -> [w204 _]
          frame False {
          }
          frame True {
            n73 = Unbundle By Name(w216) -> ("API Return Event"=w213:refnum<user-event>, "Tasks"=w218:T2[])
            n74 = Get Date/Time In Seconds() -> (seconds since 1Jan1904=w210:timestamp)
            n75 = Delete From Array(array=w218, index=0) -> (deleted portion=w212:T2, array with subset deleted=w215:T2[])  [unwired: 1 in]
            n76 = Bundle By Name(cluster=w212, "Task.Task State"=API_Task_State."Errored", "Task.Time Stamp"=w210, "Task.Task Error"=w209) -> (w208:T2)
            n77 = Bundle By Name(cluster=w216, "Tasks"=w215) -> (w214:T26)
            n78 = Generate User Event(user event=w213, event data cluster=w208) -> (error out=w207:errorcluster)  [unwired: 2 in, 1 out]
            n79 = flat-sequence {
              tunnel: w207 -> [_]
              frame #0 {
              }
            }
          }
        }
        n80 = call <vilib>:"Clear Errors.vi"("error in (no error)"=w200) -> ()  [unwired: 5 in, 2 out]
      }
      frame "Exit" {
        n81 = call <vilib>:"Add State(s) to Queue__JKI_lib_State_Machine.vi"("State(s) in (\"\")"=w224) -> ("States Out"=w223:string)  [unwired: 14 in]
      }
      frame "---------- Data ----------" {
        n82 = call <vilib>:"Add State(s) to Queue__JKI_lib_State_Machine.vi"("State(s) in (\"\")"=w229) -> ("States Out"=w228:string)  [unwired: 14 in]
      }
      frame "Process: Sync" {
        n83 = Unbundle By Name(w234) -> ("Process Sync"=w232:refnum<notifier>)
        n84 = Send Notification(notification=TRUE, notifier=w232, error in (no error)=w230) -> (error out=w231:errorcluster)  [unwired: 1 out]
        n85 = call <vilib>:"Add State(s) to Queue__JKI_lib_State_Machine.vi"("State(s) in (\"\")"=w237) -> ("States Out"=w236:string)  [unwired: 14 in]
      }
      frame "Data: Initialize" {
        w243 = T25 refnum  # Session out
        w247 = 0  # Move Index
        w248 = T11[] []  # Stage Moves
        w250 = variant  # Current Task. Return Value
        w251 = T4 {"Command"=enum."GetExplicitMessage", "Arguments"="", "Data"=variant}  # Current Task
        w249 = T14 {"Motor IP Addresss"="", "Current Position"=0, "Pulse_Per_mm"=0, "PrePrint"=[], "Load Position_mm"=0, "Laminate Position_mm"=0}  # Motion Controller Config Data
        w252 = refnum<k24> refnum  # .NET Refnum
        w254 = u32 0  # Task Start ms
        w258 = 100  # TO
        w259 = T2[] []  # Tasks
        w261 = T27 {"Current VI Reference"=refnum, "Close Panel on Exit?"=FALSE}  # Core
        n86 = call-dynamic "GetEvents_Motor Controller.vi"("error in (no error)"=w257, "TopLevel in"=w239) -> ("error out"=w245:errorcluster, "UserEvents"=w256:T28, "TopLevel out"=w246:refnum<class "Motor Controller.lvclass">)  [unwired: 7 in]
        n87 = Unbundle By Name(w256) -> ("API Executed Event"=w255:refnum<user-event>, "API Return Event"=w253:refnum<user-event>)
        n88 = call "SetStageMove_Status_MotorController.vi"("error in (no error)"=w245, "Motor Controller in"=w246) -> ("error out"=w244:errorcluster, "Motor Controller out"=w240:refnum<class "Motor Controller.lvclass">)  [unwired: 8 in]
        n89 = property class="TopLevel.lvclass"(reference=w242) -> ("Methods:Accessors:Digilens Config"=w241:T15)  [unwired: 1 in, 2 out]
        n90 = Bundle("Core"=w261, "Motor Controller out"=w240, "Tasks"=w259, "TO"=w258, "API Executed Event"=w255, "API Return Event"=w253, "Current Task"=w251, "Task Start ms"=w254, ".NET Refnum"=w252, "Current Task. Return Value"=w250, "Motion Controller Config Data"=w249, "Methods:Accessors:Digilens Config"=w241, "Stage Moves"=w248, "Move Index"=w247, "Session out"=w243, "Process Sync"=w238) -> (w262:T26)  [unwired: 1 in]
      }
      frame "Data: Cleanup" {
        n91 = Unbundle By Name(w268) -> ("Core.Current VI Reference"=w270:refnum<vi>, ".NET Refnum"=w266:refnum<k24>)
        n92 = Close Reference(reference=w266, error in (no error)=w264) -> (error out=w265:errorcluster)
        n93 = Close Reference(reference=w270, error in (no error)=w265) -> (error out=w269:errorcluster)
        n94 = call <vilib>:"Add State(s) to Queue__JKI_lib_State_Machine.vi"("State(s) in (\"\")"=w272) -> ("States Out"=w271:string)  [unwired: 14 in]
      }
      frame "---------- UI ----------" {
        n95 = call <vilib>:"Add State(s) to Queue__JKI_lib_State_Machine.vi"("State(s) in (\"\")"=w277) -> ("States Out"=w276:string)  [unwired: 14 in]
      }
      frame "UI: Initialize" {
        n96 = call <userlib>:"Fit VI window to Largest Dec__ogtk.vi"("error in (no error)"=w279) -> ("error out"=w278:errorcluster)  [unwired: 5 in, 1 out]
        n97 = call <vilib>:"Add State(s) to Queue__JKI_lib_State_Machine.vi"("State(s) in (\"\")"=w283) -> ("States Out"=w282:string)  [unwired: 14 in]
      }
      frame "UI: Cursor Set" {
        # "Argument"
        n98 = case shown="\"Idle\", Default" w285 {
          tunnel: w287 -> [w292 w294]
          tunnel: [w291 w293] -> w286
          frame "Idle", Default {
            n99 = call <vilib>:"Unset Busy.vi"("error in (no error)"=w292) -> ("error out"=w291:errorcluster)  [unwired: 10 in]
          }
          frame "Busy" {
            n100 = call <vilib>:"Set Busy.vi"("error in (no error)"=w294) -> ("error out"=w293:errorcluster)  [unwired: 9 in, 1 out]
          }
        }
        n101 = call <vilib>:"Add State(s) to Queue__JKI_lib_State_Machine.vi"("State(s) in (\"\")"=w290) -> ("States Out"=w289:string)  [unwired: 14 in]
      }
      frame "UI: Front Panel State" {
        # "Argument"
        n102 = Unbundle By Name(w298) -> ("Core.Current VI Reference"=w297:refnum<vi>)
        n103 = case shown="\"Open\", Default" w296 {
          tunnel: w300 -> [w306 w319]
          tunnel: [w308 w320] -> w299
          tunnel: w297 -> [w307 w317]
          frame "Open", Default {
            n104 = property class="VI"(reference=w307, error in=w306) -> (reference out=w304:refnum<vi>, error out=w305:errorcluster, "Front Panel.Open"=w303:bool)
            n105 = case shown="False" w303 {
              tunnel: [w311 w314] -> w308
              tunnel: w305 -> [w310 w314]
              tunnel: w304 -> [w309 _]
              frame False {
                n106 = invoke class="VI" method="FP.Open"(reference=w309, error in=w310, "Activate"=TRUE, "State"=T7."Standard") -> (error out=w311:errorcluster)  [unwired: 1 in, 4 out]
              }
              frame True {
              }
            }
          }
          frame "Close" {
            n107 = property class="VI"(reference=w317, error in=w319) -> (reference out=w316:refnum<vi>, error out=w318:errorcluster, "Front Panel.Open"=w315:bool)
            n108 = case shown="True" w315 {
              tunnel: [w321 w324] -> w320
              tunnel: w318 -> [w321 w323]
              tunnel: w316 -> [_ w322]
              frame False {
              }
              frame True {
                n109 = invoke class="VI" method="FP.Close"(reference=w322, error in=w323) -> (error out=w324:errorcluster)  [unwired: 1 in, 2 out]
              }
            }
          }
        }
        n110 = call <vilib>:"Add State(s) to Queue__JKI_lib_State_Machine.vi"("State(s) in (\"\")"=w302) -> ("States Out"=w301:string)  [unwired: 14 in]
      }
      frame "---------- Macro ----------" {
        n111 = call <vilib>:"Add State(s) to Queue__JKI_lib_State_Machine.vi"("State(s) in (\"\")"=w329) -> ("States Out"=w328:string)  [unwired: 14 in]
      }
      frame "Macro: Initialize" {
        w332 = "Data: Initialize\n/*Connection: Open\nConnectionEthIP: Open\n/*Powerup Servo\nInitialize Core Data\nUI: Initialize\nEvents: Register Events\nProcess: Sync\n/*UI: Front Panel State >> Open"  # Data: Initialize /*Connection: Open ConnectionEthIP: Open /*Powerup Servo Initialize Core Data UI: Initialize Events: Register Events Process: Sync /*UI: Front Panel State >> Open
        n112 = call <vilib>:"Add State(s) to Queue__JKI_lib_State_Machine.vi"("State(s) in (\"\")"=w332) -> ("States Out"=w333:string)  [unwired: 14 in]
      }
      frame "Macro: Exit" {
        n113 = Unbundle By Name(w342) -> ("Core.Close Panel on Exit?"=w341:bool)
        n114 = Select(t="UI: Front Panel State >> Close", s=w341, f="") -> (s? t:f=w338:string)
        n115 = call <vilib>:"Add State(s) to Queue__JKI_lib_State_Machine.vi"("State(s) in (\"\")"=w338, "State(s) at Back (\"\")"="Data: Cleanup\n/*Connection: Close\nConnectionEthIP: Close\nEvents: Unregister Events\nExit") -> ("States Out"=w336:string)  [unwired: 13 in]
        n116 = call <vilib>:"Add State(s) to Queue__JKI_lib_State_Machine.vi"("State(s) in Front (\"\")"=w336, "State(s) in (\"\")"=w345) -> ("States Out"=w344:string)  [unwired: 13 in]
      }
      frame "Macro: Stage Move Recipe" {
        n117 = call <vilib>:"Add State(s) to Queue__JKI_lib_State_Machine.vi"("State(s) in Front (\"\")"="Recipe: Stage Move\nRecipe: Check Complete", "State(s) in (\"\")"=w347) -> ("States Out"=w348:string)  [unwired: 13 in]
      }
      frame "---------- Events ----------" {
      }
      frame "Events: Register Events" {
        n118 = call-dynamic "GetEvents_TopLevel.vi"("error in (no error)"=w361, "TopLevel in"=w363) -> ("error out"=w362:errorcluster, "UserEvents"=w360:T29)  [unwired: 7 in, 1 out]
        n119 = Unbundle By Name(w360) -> ("Exit Event"=w359:refnum<user-event>)
        n120 = Unbundle By Name(w368) -> ("Motor Controller out"=w367:refnum<class "Motor Controller.lvclass">)
        n121 = call-dynamic "GetEvents_Motor Controller.vi"("error in (no error)"=w362, "TopLevel in"=w367) -> ("error out"=w366:errorcluster, "UserEvents"=w365:T28)  [unwired: 7 in, 1 out]
        n122 = Unbundle By Name(w365) -> ("API Incoming Event"=w364:refnum<user-event>, "API Executed Event"=w357:refnum<user-event>, "StopEvent"=w356:refnum<user-event>)
        n123 = register-events(w364, w357, w359, w356) -> (reference out=w369:refnum<event-registration>)  [unwired: 2 in, 1 out]
        n124 = Bundle By Name(cluster=w368, "API Executed Event"=w357) -> (w358:T26)
        n125 = call <vilib>:"Add State(s) to Queue__JKI_lib_State_Machine.vi"("State(s) in (\"\")"=w371) -> ("States Out"=w370:string)  [unwired: 14 in]
      }
      frame "Events: Unregister Events" {
        n126 = Unregister For Events(event registration refnum=w372, error in=w374) -> (error out=w373:errorcluster)
        n127 = call <vilib>:"Add State(s) to Queue__JKI_lib_State_Machine.vi"("State(s) in (\"\")"=w377) -> ("States Out"=w376:string)  [unwired: 14 in]
      }
      frame "---------- API ----------" {
      }
      frame "API: Abort" {
        n128 = Unbundle By Name(w383) -> ("Session out"=w386:T25)
        n129 = call "SendLVEthIP_ExplicitMessage.vi"("error in (no error)"=w388, "value"=1000, "Motor Controller Parameter"=Motor_Controller_Parameter-Set."Stop Stage", "Refnum in"=w386) -> ("error out"=w387:errorcluster, "Refnum out"=w382:T25)  [unwired: 6 in]
        n130 = Bundle By Name(cluster=w383, "Session out"=w382) -> (w384:T26)
      }
      frame "API: GetExplicitMessage" {
        n131 = Unbundle By Name(w407) -> ("Session out"=w393:T25, ".NET Refnum"=w406:refnum<k24>, "Current Task.Data"=w404:variant)
        n132 = Variant To Data(error in=w400, type=Motor_Controller_Parameter-Get."Print Speed" ("Motor Controller Parameter-Get"), Variant=w404) -> (data=w402:T8, error out=w401:errorcluster)
        n133 = disable-structure shown="Enabled" {
          disable-tunnel: w406 -> [w416 w423]
          disable-tunnel: [w415 w421] -> w405
          disable-tunnel: w402 -> [w414 w420]
          disable-tunnel: w401 -> [w413 w422]
          disable-tunnel: [w410 w417] -> w395
          disable-tunnel: [w409 w423] -> w394
          disable-tunnel: w393 -> [_ w419]
          disable-tunnel: [_ w418] -> w392
          frame Disabled {
            n134 = call "GetExplicitMessage.vi"("error in (no error)"=w413, "Motor Controller Parameter"=w414, ".NET Refnum in"=w416) -> ("error out"=w415:errorcluster, "GetAttributeSingle"=w411:u8[], "size"=w412:i32, ".NET Refnum out"=w409:refnum<k24>)  [unwired: 4 in, 1 out]
            n135 = Bundle("size"=w412, "GetAttributeSingle"=w411) -> (w410:cluster{"size":i32, "GetAttributeSingle":u8[]})  [unwired: 1 in]
          }
          frame Enabled {
            n136 = call "GetLVExplicitMessage.vi"("error in (no error)"=w422, "Motor Controller Parameter"=w420, "Session in"=w419) -> ("error out"=w421:errorcluster, "Session out"=w418:T25, "Data (U32)"=w417:u32)  [unwired: 5 in, 1 out]
          }
        }
        n137 = Bundle By Name(cluster=w407, "Session out"=w392, ".NET Refnum"=w394, "Current Task. Return Value"=w395) -> (w396:T26)
        n138 = call <vilib>:"Add State(s) to Queue__JKI_lib_State_Machine.vi"("State(s) in Front (\"\")"="Task: Completed", "State(s) in (\"\")"=w398) -> ("States Out"=w399:string)  [unwired: 13 in]
      }
      frame "API: SetExplicitMessage" {
        (unwired) Motor_Controller_Parameter-Set."Print Speed" ("Motor Controller Parameter")
        n139 = Unbundle By Name(w441) -> ("Session out"=w429:T25, ".NET Refnum"=w440:refnum<k24>, "Current Task.Data"=w439:variant)
        n140 = Variant To Data(error in=w437, type=T9 {"Motor Controller Parameter"=enum."Home Stage", "value"=0} ("SetExplicitMessage API Data"), Variant=w439) -> (data=w431:T9, error out=w438:errorcluster)
        n141 = Unbundle By Name(w431) -> ("Motor Controller Parameter"=w425:T1, "value"=w428:i32)
        n142 = case shown="\"Move Stage to Under PH1\"..\"Print Stage\"" w425 {
          tunnel: ["Task: Completed" "Check Stage Move Complete\nTask: Completed"] -> w424
          frame Default {
          }
          frame "Move Stage to Under PH1".."Print Stage" {
          }
        }
        n143 = disable-structure shown="Enabled" {
          disable-tunnel: w440 -> [w453 w460]
          disable-tunnel: [w452 w458] -> w426
          disable-tunnel: w438 -> [w451 w459]
          disable-tunnel: [w448 _] -> w433
          disable-tunnel: w425 -> [w447 w456]
          disable-tunnel: w428 -> [w446 w457]
          disable-tunnel: [w445 w460] -> w430
          disable-tunnel: w429 -> [_ w455]
          disable-tunnel: [_ w454] -> w427
          frame Disabled {
            n144 = call "SetExplicitMessage.vi"("value"=w446, "error in (no error)"=w451, "Motor Controller Parameter"=w447, ".NET Refnum in"=w453) -> ("error out"=w452:errorcluster, "GetAttributeSingle"=w449:u8[], "size"=w450:i32, ".NET Refnum out"=w445:refnum<k24>)  [unwired: 3 in, 1 out]
            n145 = Bundle("size"=w450, "GetAttributeSingle"=w449) -> (w448:cluster{"size":i32, "GetAttributeSingle":u8[]})  [unwired: 1 in]
          }
          frame Enabled {
            n146 = call "SendLVEthIP_ExplicitMessage.vi"("error in (no error)"=w459, "value"=w457, "Motor Controller Parameter"=w456, "Refnum in"=w455) -> ("error out"=w458:errorcluster, "Refnum out"=w454:T25)  [unwired: 6 in]
          }
        }
        n147 = Bundle By Name(cluster=w441, "Session out"=w427, ".NET Refnum"=w430, "Current Task. Return Value"=w433) -> (w434:T26)
        n148 = call <vilib>:"Add State(s) to Queue__JKI_lib_State_Machine.vi"("State(s) in Front (\"\")"=w424, "State(s) in (\"\")"=w435) -> ("States Out"=w436:string)  [unwired: 13 in]
      }
      frame "Check Stage Move Complete" {
        n149 = Unbundle By Name(w479) -> ("Session out"=w467:T25, "Current Task.Data"=w478:variant)
        n150 = Variant To Data(error in=w477, type=T9 {"Motor Controller Parameter"=enum."Home Stage", "value"=0} ("SetExplicitMessage API Data"), Variant=w478) -> (data=w472:T9, error out=w468:errorcluster)
        n151 = Unbundle By Name(w472) -> ("Motor Controller Parameter"=w471:T1, "value"=w470:i32)
        n152 = case shown="\"Move Stage to Under PH1\"..\"Print Stage\"" w471 {
          tunnel: w470 -> [_ w491]
          tunnel: w467 -> [w482 w494]
          tunnel: w468 -> [w483 w493]
          tunnel: [w483 w492] -> w469
          tunnel: [w482 w490] -> w466
          tunnel: [TRUE w486] -> w465
          tunnel: [_ w484] -> w461
          frame Default {
          }
          frame "Move Stage to Under PH1".."Print Stage" {
            n153 = call "GetLVExplicitMessage.vi"("error in (no error)"=w493, "Motor Controller Parameter"=Motor_Controller_Parameter-Get."PR Path", "Session in"=w494) -> ("error out"=w492:errorcluster, "Session out"=w490:T25, "Data (U32)"=w485:u32)  [unwired: 5 in, 1 out]
            n154 = Add(x=u32 20000, y=w491) -> (x+y=w487:u32)
            n155 = To Variant(anything=w485) -> (Variant=w484:variant)
            n156 = Equal?(x=w487, y=w485) -> (x = y?=w486:bool)
          }
        }
        n157 = Bundle By Name(cluster=w479, "Session out"=w466, "Current Task. Return Value"=w461) -> (w474:T26)
        n158 = Select(t="", s=w465, f="Idle\nCheck Stage Move Complete") -> (s? t:f=w462:string)
        n159 = call <vilib>:"Add State(s) to Queue__JKI_lib_State_Machine.vi"("State(s) in Front (\"\")"=w462, "State(s) in (\"\")"=w475) -> ("States Out"=w476:string)  [unwired: 13 in]
      }
      frame "API: Execute Stage Move Recipe" {
        n160 = Unbundle By Name(w505) -> ("Current Task.Data"=w504:variant)
        n161 = Variant To Data(error in=w503, type=path "", Variant=w504) -> (data=w498:path, error out=w497:errorcluster)
        n162 = Format Into String(format string="Recipe: Read XML>>%s\nMacro: Stage Move Recipe", error in=w497, w498) -> (resulting string=w495:string, error out=w496:errorcluster)  [unwired: 1 in]
        n163 = call <vilib>:"Add State(s) to Queue__JKI_lib_State_Machine.vi"("State(s) in Front (\"\")"=w495, "State(s) in (\"\")"=w500) -> ("States Out"=w501:string)  [unwired: 13 in]
      }
      frame "API: Read Stage Move Recipe" {
        n164 = Unbundle By Name(w517) -> ("Current Task.Data"=w516:variant)
        n165 = Variant To Data(error in=w515, type=path "", Variant=w516) -> (data=w510:path, error out=w509:errorcluster)
        n166 = Format Into String(format string="Recipe: Read XML>>%s", error in=w509, w510) -> (resulting string=w507:string, error out=w508:errorcluster)  [unwired: 1 in]
        n167 = call <vilib>:"Add State(s) to Queue__JKI_lib_State_Machine.vi"("State(s) in Front (\"\")"=w507, "State(s) in (\"\")"=w512) -> ("States Out"=w513:string)  [unwired: 13 in]
      }
      frame "---------- Tasks ----------" {
      }
      frame "Task: Completed" {
        n168 = Unbundle By Name(w529) -> ("API Executed Event"=w527:refnum<user-event>, "Tasks"=w526:T2[], "Current Task. Return Value"=w523:variant)
        n169 = Empty Array?(array=w526) -> (empty?=w528:bool)
        n170 = case shown="False" w528 {
          tunnel: w527 -> [w538 _]
          tunnel: w526 -> [w539 _]
          tunnel: w524 -> [w536 w540]
          tunnel: [w535 w540] -> w525
          tunnel: w523 -> [w533 _]
          frame False {
            n171 = Index Array(array=w539) -> (element=w537:T2)  [unwired: 1 in]
            n172 = Bundle By Name(cluster=w537, "Task.Task State"=API_Task_State."Completed", "Return Value"=w533) -> (w534:T2)
            n173 = Generate User Event(user event=w538, event data cluster=w534, error in=w536) -> (error out=w535:errorcluster)  [unwired: 1 in, 1 out]
          }
          frame True {
          }
        }
      }
      frame "Task: Check Timeout" {
        n174 = Unbundle By Name(w549) -> ("API Executed Event"=w547:refnum<user-event>, "Task Start ms"=w542:u32, "Tasks"=w544:T2[], "Motor Controller out"=w541:refnum<class "Motor Controller.lvclass">)
        n175 = Index Array(array=w544) -> (element=w543:T2)  [unwired: 1 in]
        n176 = Empty Array?(array=w544) -> (empty?=w548:bool)
        n177 = case shown="True" w548 {
          tunnel: w547 -> [w553 _]
          tunnel: w545 -> [w559 w568]
          tunnel: [w554 w569] -> w546
          tunnel: w543 -> [w558 _]
          tunnel: w542 -> [w562 _]
          tunnel: w541 -> [_ w570]
          frame False {
            n178 = Unbundle By Name(w558) -> ("Task.Timeout (ms)"=w560:u32)
            n179 = Tick Count (ms)() -> (millisecond timer value=w552:u32)
            n180 = Subtract(x=w552, y=w562) -> (x-y=w561:u32)
            n181 = Bundle By Name(cluster=w558, "Task.Task State"=API_Task_State."Errored") -> (w556:T2)
            n182 = Greater Or Equal?(x=w561, y=w560) -> (x >= y?=w555:bool)
            n183 = case shown="False" w555 {
              tunnel: w559 -> [w563 w567]
              tunnel: w556 -> [_ w565]
              tunnel: [w563 w566] -> w554
              tunnel: w553 -> [_ w564]
              frame False {
              }
              frame True {
                n184 = Generate User Event(user event=w564, event data cluster=w565, error in=w567) -> (error out=w566:errorcluster)  [unwired: 1 in, 1 out]
              }
            }
          }
          frame True {
            n185 = disable-structure shown="Enabled" {
              disable-tunnel: w570 -> [w573 _]
              disable-tunnel: [w572 w575] -> w569
              disable-tunnel: w568 -> [w571 w575]
              frame Enabled {
                n186 = call "SetStageBusy_Status_MotorController.vi"("error in (no error)"=w571, "Stage Busy?"=FALSE, "Motor Controller in"=w573) -> ("error out"=w572:errorcluster)  [unwired: 7 in, 1 out]
              }
              frame Disabled {
              }
            }
          }
        }
      }
      frame "Task: Check Pending" {
        n187 = Unbundle By Name(w577) -> ("API Executed Event"=w586:refnum<user-event>, "Task Start ms"=w583:u32, "Tasks"=w582:T2[], "Motor Controller out"=w576:refnum<class "Motor Controller.lvclass">)
        n188 = Empty Array?(array=w582) -> (empty?=w587:bool)
        n189 = case shown="False" w587 {
          tunnel: w586 -> [_ _]
          tunnel: w584 -> [w597 w605]
          tunnel: [w595 w606] -> w585
          tunnel: w583 -> [_ _]
          tunnel: w582 -> [w604 _]
          tunnel: [w594 _] -> w579
          tunnel: w577 -> [w593 w608]
          tunnel: [w591 w608] -> w578
          tunnel: w576 -> [_ w607]
          frame False {
            n190 = Index Array(array=w604) -> (element=w599:T2)  [unwired: 1 in]
            n191 = Unbundle By Name(w599) -> ("Command"=w598:variant)
            n192 = Tick Count (ms)() -> (millisecond timer value=w592:u32)
            n193 = Variant To Data(error in=w597, type=T4 {"Command"=enum."GetExplicitMessage", "Arguments"="", "Data"=variant} ("API Command Cluster"), Variant=w598) -> (data=w589:T4, error out=w596:errorcluster)
            n194 = Unbundle By Name(w589) -> ("Command"=w601:T5, "Arguments"=w600:string)
            n195 = Bundle By Name(cluster=w593, "TO"=100, "Task Start ms"=w592, "Current Task"=w589) -> (w591:T26)
            n196 = Format Into String(format string="API: %s>>%s", error in=w596, w601, w600) -> (resulting string=w594:string, error out=w595:errorcluster)  [unwired: 1 in]
          }
          frame True {
            n197 = disable-structure shown="Enabled" {
              disable-tunnel: w607 -> [w611 _]
              disable-tunnel: [w610 w613] -> w606
              disable-tunnel: w605 -> [w609 w613]
              frame Enabled {
                n198 = call "SetStageBusy_Status_MotorController.vi"("error in (no error)"=w609, "Stage Busy?"=FALSE, "Motor Controller in"=w611) -> ("error out"=w610:errorcluster)  [unwired: 7 in, 1 out]
              }
              frame Disabled {
              }
            }
          }
        }
        n199 = call <vilib>:"Add State(s) to Queue__JKI_lib_State_Machine.vi"("State(s) in Front (\"\")"=w579, "State(s) in (\"\")"=w580) -> ("States Out"=w581:string)  [unwired: 13 in]
      }
      frame "Task: Remove on Error" {
        n200 = Unbundle By Name(w621) -> ("Motor Controller out"=w614:refnum<class "Motor Controller.lvclass">, "API Return Event"=w623:refnum<user-event>, "Tasks"=w622:T2[])
        n201 = for {
          tunnel: w623 -> [w638]
          tunnel: w622 -> [w637] mode=indexing
          shift-right: [w632] -> w616
          shift-left: w620 -> [w633]
          n202 = Get Date/Time In Seconds() -> (seconds since 1Jan1904=w634:timestamp)
          n203 = Bundle By Name(cluster=w637, "Task.Task State"=API_Task_State."Errored", "Task.Time Stamp"=w634) -> (w636:T2)
          n204 = Generate User Event(user event=w638, event data cluster=w636, error in=w633) -> (error out=w632:errorcluster)  [unwired: 1 in, 1 out]
        }
        n205 = Bundle By Name(cluster=w621, "TO"=100, "Tasks"=T2[] []) -> (w619:T26)
        n206 = disable-structure shown="Enabled" {
          disable-tunnel: w614 -> [w629 _]
          disable-tunnel: [w628 w631] -> w615
          disable-tunnel: w616 -> [w627 w631]
          frame Enabled {
            n207 = call "SetStageBusy_Status_MotorController.vi"("error in (no error)"=w627, "Stage Busy?"=FALSE, "Motor Controller in"=w629) -> ("error out"=w628:errorcluster)  [unwired: 7 in, 1 out]
          }
          frame Disabled {
          }
        }
        n208 = call <vilib>:"Add State(s) to Queue__JKI_lib_State_Machine.vi"("State(s) in (\"\")"=w624) -> ("States Out"=w625:string)  [unwired: 14 in]
      }
      frame "-----------Ethernet IP Communication-----------" {
      }
      frame "ConnectionEthIP: Open" {
        # "Should Come from Config"
        n209 = call <vilib>:"EthernetIP Open Session.vi"("error in"=w645, "Session in"="192.168.1.12" ("String")) -> ("error out"=w646:errorcluster, "Session out"=w648:T25)  [unwired: 8 in]
        n210 = Bundle By Name(cluster=w643, "Session out"=w648) -> (w644:T26)
      }
      frame "ConnectionEthIP: Close" {
        n211 = Unbundle By Name(w653) -> ("Session out"=w654:T25)
        n212 = call <vilib>:"EthernetIP Close Session.vi"("error in"=w651, "Session in"=w654) -> ("error out"=w652:errorcluster)  [unwired: 9 in]
      }
      frame "Connection: Open" {
        # "Should Come from Config"
        n213 = call "OpenEthernetIPConnection.vi"("String"="192.168.1.12") -> ("error out"=w659:errorcluster, ".NET Refnum out"=w657:refnum<k24>)  [unwired: 9 in]
        n214 = Bundle By Name(cluster=w663, ".NET Refnum"=w657) -> (w658:T26)
        n215 = Merge Errors(w665, w659) -> (w660:errorcluster)
      }
      frame "Connection: Close" {
        n216 = Unbundle By Name(w667) -> (".NET Refnum"=w666:refnum<k24>)
        n217 = call "CloseEthernetIP connection.vi"("error in (no error)"=w669, ".NET Refnum in"=w666) -> ("error out"=w668:errorcluster)  [unwired: 9 in]
      }
      frame "------------Servo-----------" {
      }
      frame "Powerup Servo" {
        # "Check the output and updated enabled? flag in status to update it in the UI"
        n218 = Unbundle By Name(w684) -> ("Session out"=w678:T25, ".NET Refnum"=w683:refnum<k24>)
        n219 = disable-structure shown="Enabled" {
          disable-tunnel: w683 -> [w691 _]
          disable-tunnel: [w690 w696] -> w682
          disable-tunnel: w681 -> [w689 w697]
          disable-tunnel: Motor_Controller_Parameter-Set."Enable Servo" ("Motor Controller Parameter") -> [w688 w694]
          disable-tunnel: 1 ("value") -> [w687 w695]
          disable-tunnel: w678 -> [_ w693]
          disable-tunnel: [_ w692] -> w676
          frame Disabled {
            n220 = call "SetExplicitMessage.vi"("value"=w687, "error in (no error)"=w689, "Motor Controller Parameter"=w688, ".NET Refnum in"=w691) -> ("error out"=w690:errorcluster)  [unwired: 3 in, 4 out]
          }
          frame Enabled {
            n221 = call "SendLVEthIP_ExplicitMessage.vi"("error in (no error)"=w697, "value"=w695, "Motor Controller Parameter"=w694, "Refnum in"=w693) -> ("error out"=w696:errorcluster, "Refnum out"=w692:T25)  [unwired: 6 in]
          }
        }
        n222 = Bundle By Name(cluster=w684, "Session out"=w676) -> (w677:T26)
      }
      frame "----------Recipe------------" {
      }
      frame "Recipe: Read XML" {
        w717 = T30 {"Batch_Move"=[]} ("Recipe")
        n223 = String To Path(string=w721) -> (path=w720:path)
        n224 = call <vilib>:"Easy Read XML File__JKI EasyXML.vi"("error in (no error)"=w719, "LabVIEW Data (Type)"=w717, "XML File Path"=w720) -> ("error out"=w716:errorcluster, "LabVIEW Data"=w718:variant)  [unwired: 6 in, 1 out]
        n225 = Variant To Data(error in=w716, type=w717, Variant=w718) -> (data=w715:T30, error out=w712:errorcluster)
        n226 = Unbundle By Name(w715) -> ("Batch_Move"=w714:T31)
        n227 = for {
          tunnel: w714 -> [w727] mode=indexing
          tunnel: [w723] -> w706 mode=concatenating
          i -> [w724]
          n228 = Unbundle By Name(w727) -> ("Cycles"=w725:u32, "Move"=w726:cluster{"Index_mm":i32, "Speed_mm_s":i32}[])
          n229 = for {
            N: w725 -> [_]
            tunnel: w726 -> [w730]
            tunnel: w724 -> [w732]
            tunnel: [w728] -> w723 mode=concatenating
            i -> [w731]
            n230 = Format Into String(format string="Batch_Move %d : Cycle %d", w732, w731) -> (resulting string=w729:string)  [unwired: 2 in, 1 out]
            n231 = for {
              tunnel: w730 -> [w736] mode=indexing
              tunnel: w729 -> [w737]
              tunnel: [w735] -> w728 mode=indexing
              n232 = Bundle By Name(cluster=T11 {"Batch & Cycle"="", "Move"={"Index_mm"=0, "Speed_mm_s"=0}, "Status"=enum."Pending"} ("Move Data"), "Move"=w736, "Batch & Cycle"=w737) -> (w735:T11)
            }
          }
        }
        n233 = Unbundle By Name(w709) -> ("Motor Controller out"=w713:refnum<class "Motor Controller.lvclass">)
        n234 = Bundle By Name(cluster=w709, "Move Index"=0, "Stage Moves"=w706) -> (w710:T26)
        n235 = Bundle By Name(cluster=T10 {"Current Step"="", "Move Data"=[]} ("Stage Moves"), "Move Data"=w706) -> (w705:T10)
        n236 = call "SetStageMove_Status_MotorController.vi"("error in (no error)"=w712, "Stage Moves"=w705, "Motor Controller in"=w713) -> ("error out"=w711:errorcluster)  [unwired: 7 in, 1 out]
        n237 = call <vilib>:"Add State(s) to Queue__JKI_lib_State_Machine.vi"("State(s) in Front (\"\")"="Task: Completed", "State(s) in (\"\")"=w703) -> ("States Out"=w704:string)  [unwired: 13 in]
      }
      frame "Recipe: Stage Move" {
        w752 = Motor_Controller_Parameter-Set."PR Path" ("Motor Controller Parameter")
        # "Conversion done in SendLVEthIP_ExplicitMessage.vi"
        n238 = Unbundle By Name(w771) -> ("Stage Moves"=w763:T11[], "Move Index"=w762:i32, ".NET Refnum"=w770:refnum<k24>, "Session out"=w741:T25, "Motor Controller out"=w757:refnum<class "Motor Controller.lvclass">)
        n239 = Index Array(array=w763, index=w762) -> (element=w761:T11)
        n240 = Unbundle By Name(w761) -> ("Move.Speed_mm_s"=w764:i32, "Move.Index_mm"=w765:i32, "Batch & Cycle"=w747:string)
        n241 = Bundle By Name(cluster=w761, "Status"=Move_Status."In Progress") -> (w759:T11)
        n242 = Replace Array Subset(array=w763, new element=w759, index=w762) -> (w745:T11[])
        n243 = disable-structure shown="Disabled" {
          disable-tunnel: w765 -> [w785 w787]
          disable-tunnel: w764 -> [w784 w786]
          disable-tunnel: [w779 w787] -> w743
          disable-tunnel: [w774 w786] -> w742
          frame Disabled {
            n244 = Divide(x=w785, y=12.7) -> (x/y=w783:dbl)
            n245 = Multiply(x=w783, y=100000.0 ("x")) -> (x*y=w781:dbl)
            n246 = To Long Integer(number=w781) -> (32bit integer=w779:i32)
            n247 = Multiply(x=w784, y=60 ("x")) -> (x*y=w778:i32)
            n248 = Divide(x=w778, y=12.7) -> (x/y=w776:dbl)
            n249 = To Long Integer(number=w776) -> (32bit integer=w774:i32)
          }
          frame Enabled {
          }
        }
        n250 = Bundle By Name(cluster=w771, "Stage Moves"=w745) -> (w758:T26)
        n251 = Bundle By Name(cluster=T10 {"Current Step"="", "Move Data"=[]} ("Stage Move"), "Current Step"=w747, "Move Data"=w745) -> (w746:T10)
        n252 = call "SetStageMove_Status_MotorController.vi"("error in (no error)"=w755, "Stage Moves"=w746, "Motor Controller in"=w757) -> ("error out"=w756:errorcluster)  [unwired: 7 in, 1 out]
        n253 = disable-structure shown="Enabled" {
          disable-tunnel: w770 -> [w836 w843]
          disable-tunnel: Motor_Controller_Parameter-Set."Write Index" ("Motor Controller Parameter") -> [w835 w839]
          disable-tunnel: [w834 w843] -> w768
          disable-tunnel: [w833 w841] -> w766
          disable-tunnel: w756 -> [w832 w842]
          disable-tunnel: w743 -> [w831 w838]
          disable-tunnel: w741 -> [_ w840]
          disable-tunnel: [_ w837] -> w740
          frame Disabled {
            n254 = call "SetExplicitMessage.vi"("value"=w831, "error in (no error)"=w832, "Motor Controller Parameter"=w835, ".NET Refnum in"=w836) -> ("error out"=w833:errorcluster, ".NET Refnum out"=w834:refnum<k24>)  [unwired: 3 in, 3 out]
          }
          frame Enabled {
            n255 = call "SendLVEthIP_ExplicitMessage.vi"("error in (no error)"=w842, "value"=w838, "Motor Controller Parameter"=w839, "Refnum in"=w840) -> ("error out"=w841:errorcluster, "Refnum out"=w837:T25)  [unwired: 6 in]
          }
        }
        n256 = disable-structure shown="Enabled" {
          disable-tunnel: w768 -> [w823 w830]
          disable-tunnel: Motor_Controller_Parameter-Set."Write Speed" ("Motor Controller Parameter") -> [w822 w828]
          disable-tunnel: w766 -> [w821 w824]
          disable-tunnel: [w820 w830] -> w754
          disable-tunnel: [w819 w829] -> w750
          disable-tunnel: w742 -> [w818 w827]
          disable-tunnel: w740 -> [_ w826]
          disable-tunnel: [_ w825] -> w739
          frame Disabled {
            n257 = call "SetExplicitMessage.vi"("value"=w818, "error in (no error)"=w821, "Motor Controller Parameter"=w822, ".NET Refnum in"=w823) -> ("error out"=w819:errorcluster, ".NET Refnum out"=w820:refnum<k24>)  [unwired: 3 in, 3 out]
          }
          frame Enabled {
            n258 = call "SendLVEthIP_ExplicitMessage.vi"("error in (no error)"=w824, "value"=w827, "Motor Controller Parameter"=w828, "Refnum in"=w826) -> ("error out"=w829:errorcluster, "Refnum out"=w825:T25)  [unwired: 6 in]
          }
        }
        n259 = disable-structure shown="Enabled" {
          disable-tunnel: w754 -> [w810 w817]
          disable-tunnel: [w809 w817] -> w753
          disable-tunnel: w752 -> [w808 w814]
          disable-tunnel: [w807 w815] -> w751
          disable-tunnel: w750 -> [w806 w816]
          disable-tunnel: 10 ("value") -> [w805 w813]
          disable-tunnel: w739 -> [_ w812]
          disable-tunnel: [_ w811] -> w738
          frame Disabled {
            n260 = call "SetExplicitMessage.vi"("value"=w805, "error in (no error)"=w806, "Motor Controller Parameter"=w808, ".NET Refnum in"=w810) -> ("error out"=w807:errorcluster, ".NET Refnum out"=w809:refnum<k24>)  [unwired: 3 in, 3 out]
          }
          frame Enabled {
            n261 = call "SendLVEthIP_ExplicitMessage.vi"("error in (no error)"=w816, "value"=w813, "Motor Controller Parameter"=w814, "Refnum in"=w812) -> ("error out"=w815:errorcluster, "Refnum out"=w811:T25)  [unwired: 6 in]
          }
        }
        n262 = disable-structure shown="Enabled" {
          disable-tunnel: w753 -> [w793 _]
          disable-tunnel: w752 -> [w792 _]
          disable-tunnel: w751 -> [w791 w804]
          disable-tunnel: [w790 w804] -> w749
          disable-tunnel: w738 -> [w788 _]
          frame Disabled {
            n263 = disable-structure shown="Enabled" {
              disable-tunnel: w793 -> [w798 _]
              disable-tunnel: w792 -> [w797 w800]
              disable-tunnel: w791 -> [w796 w803]
              disable-tunnel: [w795 w802] -> w790
              disable-tunnel: 0 ("value") -> [w794 w801]
              disable-tunnel: w788 -> [_ w799]
              frame Disabled {
                n264 = call "SetExplicitMessage.vi"("value"=w794, "error in (no error)"=w796, "Motor Controller Parameter"=w797, ".NET Refnum in"=w798) -> ("error out"=w795:errorcluster)  [unwired: 3 in, 4 out]
              }
              frame Enabled {
                n265 = call "SendLVEthIP_ExplicitMessage.vi"("error in (no error)"=w803, "value"=w801, "Motor Controller Parameter"=w800, "Refnum in"=w799) -> ("error out"=w802:errorcluster)  [unwired: 6 in, 1 out]
              }
            }
          }
          frame Enabled {
          }
        }
      }
      frame "Recipe: Set Completed" {
        n266 = Unbundle By Name(w857) -> ("Stage Moves"=w856:T11[], "Move Index"=w855:i32, "Motor Controller out"=w851:refnum<class "Motor Controller.lvclass">)  [unwired: 1 out]
        n267 = Index Array(array=w856, index=w855) -> (element=w847:T11)
        n268 = Unbundle By Name(w847) -> ("Batch & Cycle"=w846:string)
        n269 = Bundle By Name(cluster=w847, "Status"=Move_Status."Completed") -> (w853:T11)
        n270 = Replace Array Subset(array=w856, new element=w853, index=w855) -> (w845:T11[])
        n271 = Bundle By Name(cluster=T10 {"Current Step"="", "Move Data"=[]} ("Stage Moves"), "Move Data"=w845, "Current Step"=w846) -> (w844:T10)
        n272 = Bundle By Name(cluster=w857, "Stage Moves"=w845) -> (w852:T26)
        n273 = call "SetStageMove_Status_MotorController.vi"("error in (no error)"=w850, "Stage Moves"=w844, "Motor Controller in"=w851) -> ("error out"=w849:errorcluster)  [unwired: 7 in, 1 out]
      }
      frame "Recipe: Check Complete" {
        n274 = Unbundle By Name(w878) -> ("Stage Moves"=w873:T11[], "Move Index"=w872:i32, ".NET Refnum"=w877:refnum<k24>, "Session out"=w860:T25)
        n275 = disable-structure shown="Enabled" {
          disable-tunnel: w877 -> [w884 _]
          disable-tunnel: Motor_Controller_Parameter-Get."PR Path" ("Motor Controller Parameter") -> [w883 w887]
          disable-tunnel: [w882 w890] -> w875
          disable-tunnel: w874 -> [w881 w889]
          disable-tunnel: [w880 w886] -> w861
          disable-tunnel: w860 -> [_ w888]
          disable-tunnel: [_ w885] -> _
          frame Disabled {
            n276 = call "GetExplicitMessage.vi"("error in (no error)"=w881, "Motor Controller Parameter"=w883, ".NET Refnum in"=w884) -> ("error out"=w882:errorcluster, "Data (U32)"=w880:u32)  [unwired: 4 in, 3 out]
          }
          frame Enabled {
            n277 = call "GetLVExplicitMessage.vi"("error in (no error)"=w889, "Motor Controller Parameter"=w887, "Session in"=w888) -> ("error out"=w890:errorcluster, "GetAttributeSingle"=w885:u8[], "Data (U32)"=w886:u32)  [unwired: 5 in, 1 out]
          }
        }
        n278 = Index Array(array=w873, index=w872) -> (element=w871:T11)
        n279 = Unbundle By Name(w871) -> ()  [unwired: 1 out]
        n280 = Add(x=u32 20000, y=u32 10) -> (x+y=w869:u32)
        n281 = Equal?(x=w869, y=w861) -> (x = y?=w868:bool)
        n282 = Select(t="Recipe: Set Completed\nRecipe: Check Next", s=w868, f="Idle\nRecipe: Check Complete") -> (s? t:f=w863:string)
        n283 = call <vilib>:"Add State(s) to Queue__JKI_lib_State_Machine.vi"("State(s) in Front (\"\")"=w863, "State(s) in (\"\")"=w866) -> ("States Out"=w867:string)  [unwired: 13 in]
      }
      frame "Recipe: Check Next" {
        n284 = Unbundle By Name(w897) -> ("Move Index"=w900:i32, "Stage Moves"=w902:T11[])
        n285 = Array Size(array=w902) -> (size(s)=w901:i32)
        n286 = Increment(x=w900) -> (x+1=w899:i32)
        n287 = Greater Or Equal?(x=w900, y=w901) -> (x >= y?=w894:bool)
        n288 = Bundle By Name(cluster=w897, "Move Index"=w899) -> (w898:T26)
        n289 = Select(t="Task: Completed", s=w894, f="Macro: Stage Move Recipe") -> (s? t:f=w891:string)
        n290 = call <vilib>:"Add State(s) to Queue__JKI_lib_State_Machine.vi"("State(s) in Front (\"\")"=w891, "State(s) in (\"\")"=w895) -> ("States Out"=w896:string)  [unwired: 13 in]
      }
    }
  }
  "error out" <- w3
  "Motor Controller out" <- "Motor Controller in"
